vi "Text control 2 v1.3.vi"() -> ()   [LabVIEW 2016]
panel:
  in  "Serial Settings:Serial End Mode for Reads":u16(ring)=2 items=["None", "LastBit", "TermChar"]
  in  "bytes to read":u32=5
  in  "Timeout (ms)":u32=10000
  in  "Enable Termination\nChar (T)":bool=TRUE
  in  "Termination char\n(0xA = '\\n' = LF)\n(0xD = '\\r' = CR)":u8=13 format="%.0x"
  in  "flow control":u16(ring) items=["None"=0, "XON/XOFF"=1, "RTS/CTS"=2, "DTR/DSR"=4]
  in  "stop bits":u16(ring)=10 items=["1.0"=10, "1.5"=15, "2.0"=20]
  in  "parity":u16(ring) items=["None", "Odd", "Even", "Mark", "Space"]
  in  "data bits":u16=8 min=5 max=8 step=1
  in  "VISA resource name":refnum<visa-resource-name>="COM8"
  in  "baud rate":u32=9600
  out "Serial output":string
  out "error out":errorcluster
  in  "Units":bool
  out "Elapsed Time":dbl caption="Elapsed Time (s)"
  out "Ion vs time":cluster{"Y data in":dbl[], "X data in":dbl[]}[](graph)
  out "Ig":dbl format="%.2e"
  out "Id":dbl format="%.2e"
  out "Is":dbl format="%.2e"
  out "I vs Vg":cluster{"Y data in":dbl[], "X data in":dbl[]}[](graph)
  in  "Panel Controls 2":T1={"Emergency Stop"=refnum, "TransGraph Max"=1e-05, "Text/Graph (text=false)"=TRUE, "TransGraph Min"=1e-11} {"TransGraph Min" format="%.2e"; "TransGraph Max" format="%.2e"}
  out "Currently running:":string="#output s 0 0 0 -0.008 0.008 0.002"
  in  "Lines left to run:":string
  in  "Standby":T2
  in  "Full Reset":bool
  in  "SMU4":cluster{"on/off":bool, "Voltage":dbl} {"Voltage" min=-100.0 max=100.0 format="%.2f"}
  in  "Source/Drain Range":u8(slide)=6 max=11 scale=0.0..11.0
  in  "Source/Drain\nRange mode":u16(ring) items=["Auto", "Limited", "Fixed"]
  in  "Gate Range":u8(slide)=6 max=11 scale=0.0..11.0
  in  "Gate Range\nmode":u16(ring) items=["Auto", "Limited", "Fixed"]
  in  "Gate":T3={"Gate Start"=0.0, "Gate Stop"=2.0, "Gate Step (linear only)"=1.0, "Gate Compliance"=0.0001, "Gate PComp"=0.0, "Range mode"=0, "Range"=6} {"Range" max=11 scale=0.0..11.0; "Range mode" items=["Auto", "Limited", "Fixed"]; "Gate PComp" format="%^.2e"; "Gate Compliance" format="%^.2e"; "Gate Step (linear only)" format="%^.4e"; "Gate Stop" format="%^.4e"; "Gate Start" format="%^.4e"}
  in  "Drain 2":T4={"Drain Start"=0.0, "Drain Stop"=2.0, "Drain Compliance"=0.0001, "Drain Step"=1.0, "Drain PComp"=0.0, "Range mode"=0, "Range"=6} {"Range" max=11 scale=0.0..11.0; "Range mode" items=["Auto", "Limited", "Fixed"]; "Drain PComp" format="%^.2e"; "Drain Step" format="%^.4e"; "Drain Compliance" format="%^.2e"; "Drain Stop" format="%^.4e"; "Drain Start" format="%^.4e"}
  in  "Timings 2":T5={"integration time"=0, "Short/Long integration time"=0.00064, "hold time (sec)"=0.0, "delay time (sec)"=0.0, "Step Time (0 disables)"=0.0, "sweep method"=0, "Pulse period"=0.005, "Base voltage"=0.0, "Pulse width"=0.0005} {"Pulse width" min=0.0005 max=0.1 step=0.0001 format="%.4f"; "Base voltage" format="%^.4e"; "Pulse period" min=0.005 max=1.0 step=0.0001 format="%.4f"; "sweep method" items=["Continuous", "Pulsed"]; "Step Time (0 disables)" format="%.2f"; "delay time (sec)" format="%.4f"; "hold time (sec)" format="%.4f"; "Short/Long integration time" format="%^.0e"; "integration time" scale=0.0..2.0}
  in  "Panel Controls":T6={"Emergency Stop"=refnum, "TransGraph Max"=1e-05, "Text/Graph (text=false)"=TRUE} {"TransGraph Max" format="%.2e"}
  in  "Interrupt run":bool
  in  "Drain: Compliance":dbl=0.001 format="%.8f"
  in  "Gate: Compliance":dbl=0.001 format="%.8f"
  out "Path":path=path "C:/users/rlp38/09Apr2009LTtesting/test2.txt"
  in  "hold time /s":dbl format="%.2f"
  in  "delay time /s":dbl format="%.2f"
  in  "integration time":u32(slide) max=2 step=1 scale=0.0..2.0
  in  "Integration time (short)":dbl=0.0019 min=8e-05 max=0.0019 step=8e-05 format="%^.0e"
  in  "Integration time (long)":dbl=0.32 min=0.04 max=2.0 step=0.02 format="%.2f"
  in  "Step delay /s":dbl format="%.2f"
  in  "Program":string="#pulsedstressV d 0.03 20 0 0.5 0.0827 5\n#\n#itime s\n#gaterangemode l\n#drainrangemode l\n#pulsed on 0.05 0 0.02\n#transfer d 1 -1 -0.1 -1 -1 0\n#wait-min 1\n#transfer d 1 -1 -0.1 -1 -1 0\n#output d 0 -1 -0.5 0 -1 -0.1\n#transfer d -10 40 1 5 40 35\n#transfer d -10 40 1 5 40 35\n#output d 0 40 20 0 40 1\n#\n#\n#sample 1 0.008 221 6 0.003\n#samplei 400e-6 200 6 0.002 0.1\n#vsu2pulse -10 4\n#\n#stressV 0.016 0.03 2e-4 0.1e-3 11\n#stressI 220e-7 0.08 15\n#transfer s -1 1 0.5 -0.005 0.005 0.005\n#output s 0 0 0 -0.008 0.008 0.002\n"
  # "Syntax:\nitime [s|m|l]\ngaterangemode [a|l|f]\ndrainrangemode [a|l|f]\npulsed [on|off] PulsePeriod(sec) PulseBaseVoltage PulseONWidth(sec)\nstandby [on l off]\nwait NumMilliseconds\nwait-min NumMinutes\n# texthere = comment\ntransfer [s|d] VgStart VgStop VgStep VdStart VdStop VdStep\noutput [s|d] VgStart VgStop VgStep VdStart VdStop VdStep\nsample Vg Vd NumSamples Time(s) SampleInterval(s)\nsamplei Idg NumSamples Time(s) SampleInterval(s) VDGcompliance\n# if in doubt use SampleInterval(s) = 0.004\nstressV VG VD IGcompliance IDcompliance Duration(sec)\nstressI IDG VDGcompliance Duration(sec)\nvsu2pulse Bias Duration(s)\npulsedstressV [s|d] VEstop VgON VgOFF Period(s) PulseONwidth(s) Vd\nsample-fpp Vg Vd NumSamples Time\nresample-fpp Vg Vd\ntransfer-fpp [s|d] VgStart VgStop VgStep VdStart VdStop VdStep\noutput-fpp [s|d] VgStart VgStop VgStep VdStart VdStop VdStep\nserial SerialPortCommand"
  # "Time"
  # "Sec"
  # "Min"
  # "100 samples is approx 13s with medium integration"
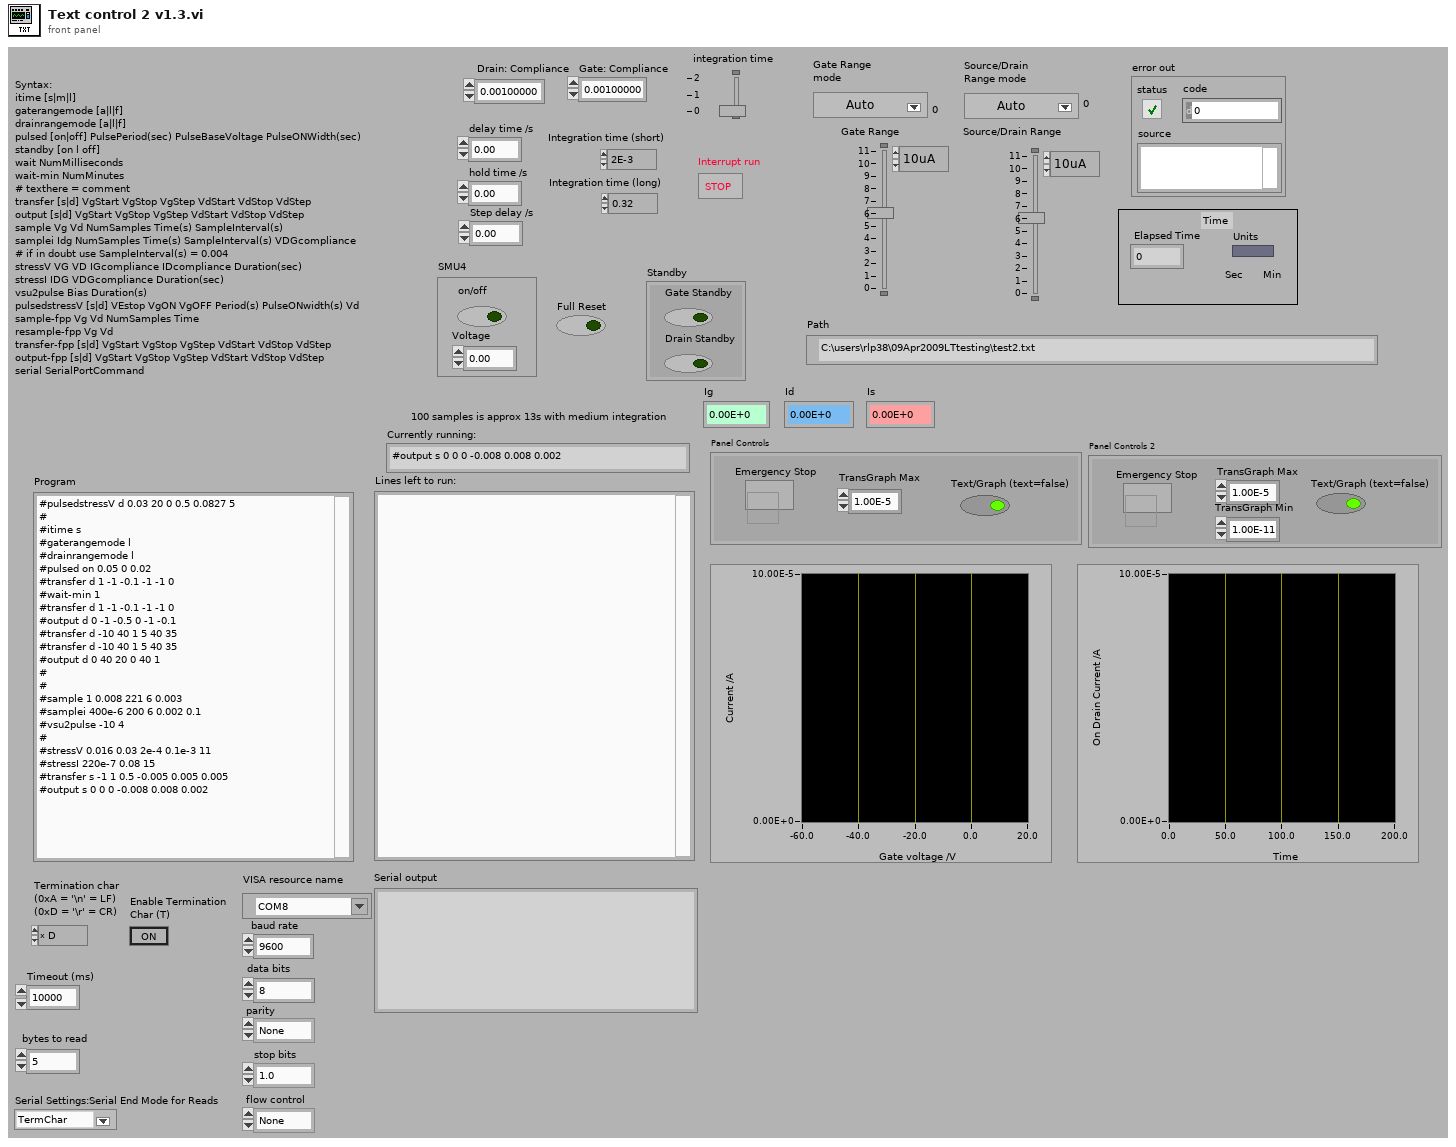
[diagram p1: front panel]
types:
  T1 = cluster{"Emergency Stop":refnum<vi>, "TransGraph Max":dbl, "Text/Graph (text=false)":bool, "TransGraph Min":dbl}
  T2 = cluster{"Gate Standby":bool, "Drain Standby":bool}
  T3 = cluster{"Gate Start":dbl, "Gate Stop":dbl, "Gate Step (linear only)":dbl, "Gate Compliance":dbl, "Gate PComp":dbl, "Range mode":u16, "Range":u8}
  T4 = cluster{"Drain Start":dbl, "Drain Stop":dbl, "Drain Compliance":dbl, "Drain Step":dbl, "Drain PComp":dbl, "Range mode":u16, "Range":u8}
  T5 = cluster{"integration time":u32, "Short/Long integration time":dbl, "hold time (sec)":dbl, "delay time (sec)":dbl, "Step Time (0 disables)":dbl, "sweep method":u16, "Pulse period":dbl, "Base voltage":dbl, "Pulse width":dbl}
  T6 = cluster{"Emergency Stop":refnum<vi>, "TransGraph Max":dbl, "Text/Graph (text=false)":bool}
  T7 = enum16{"open", "replace", "create", "open or create", "replace or create", "replace or create with confirmation"}
  T8 = cluster{"V2 Start":dbl, "V2 Step":dbl, "Number of points":i32}
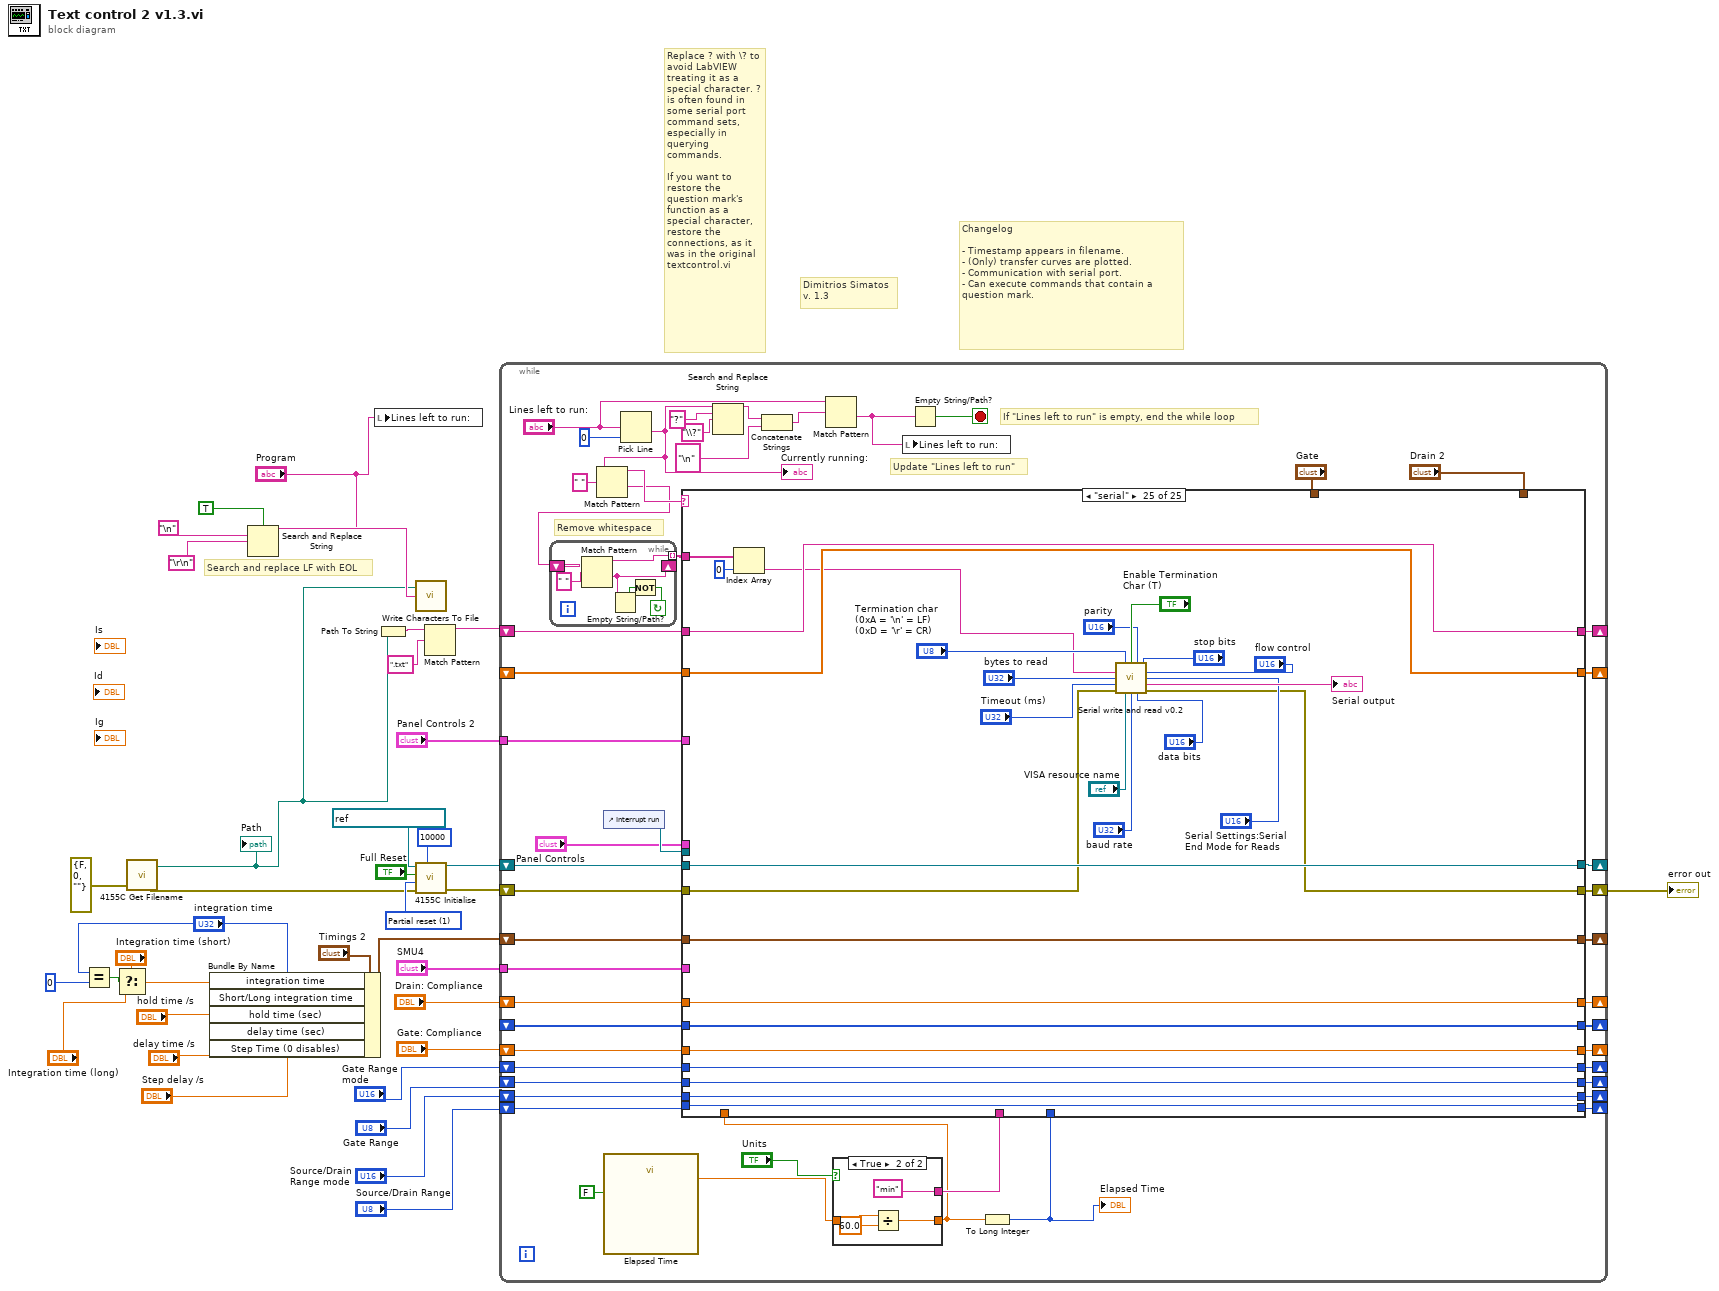
[diagram p0: block diagram]
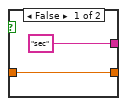
[diagram p2: hidden frame]
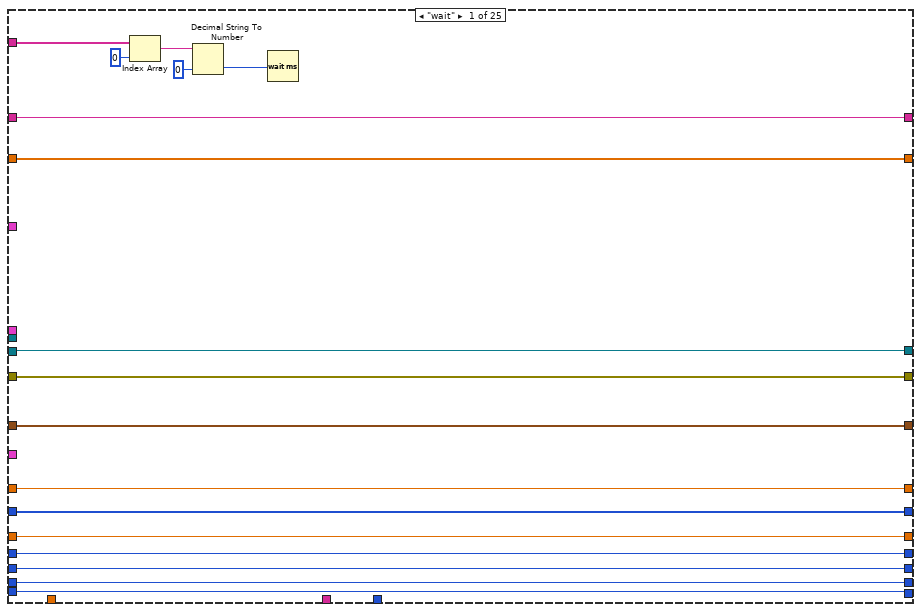
[diagram p3: hidden frame]
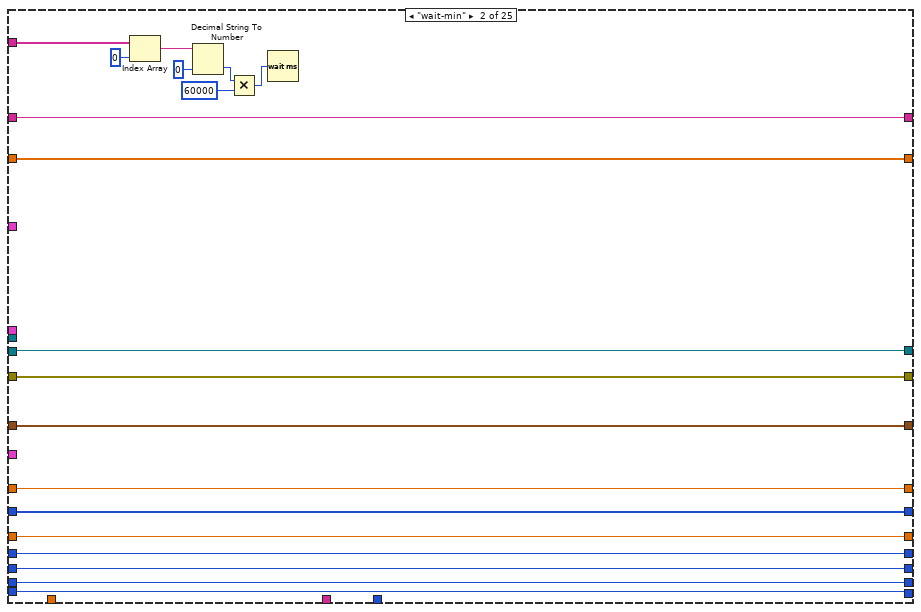
[diagram p4: hidden frame]
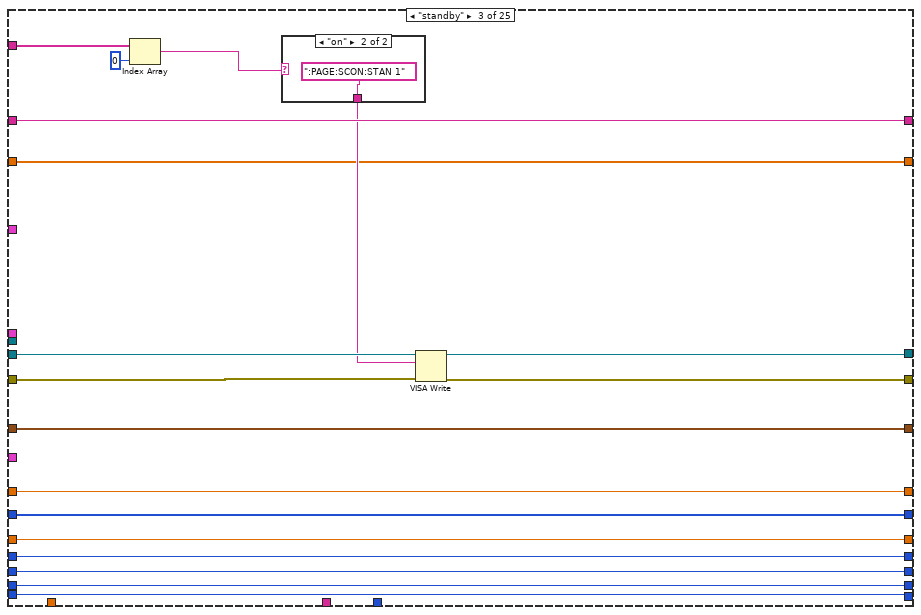
[diagram p5: hidden frame]
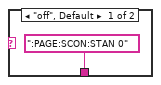
[diagram p6: hidden frame]
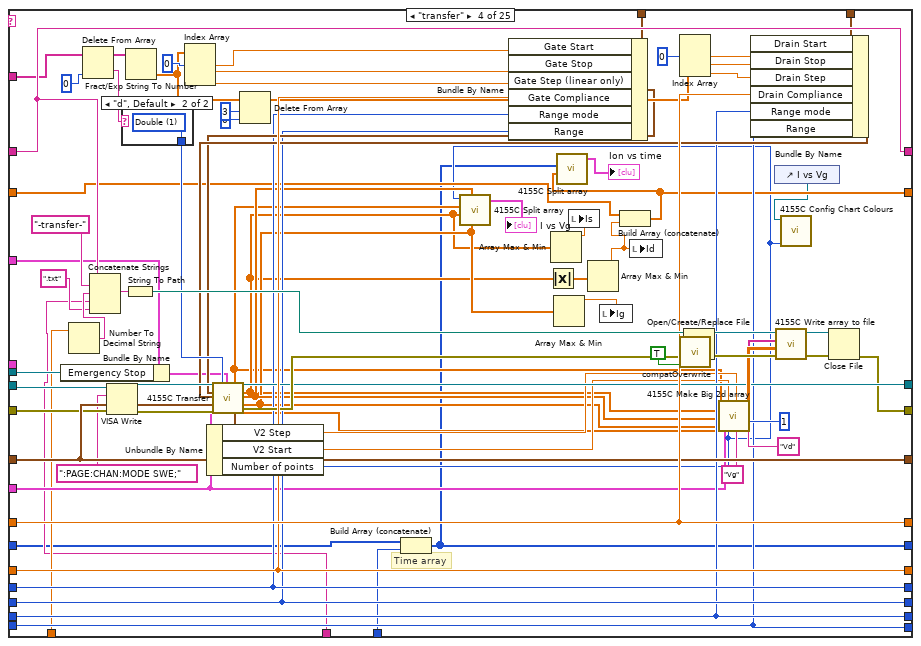
[diagram p7: hidden frame]
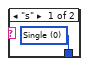
[diagram p8: hidden frame]
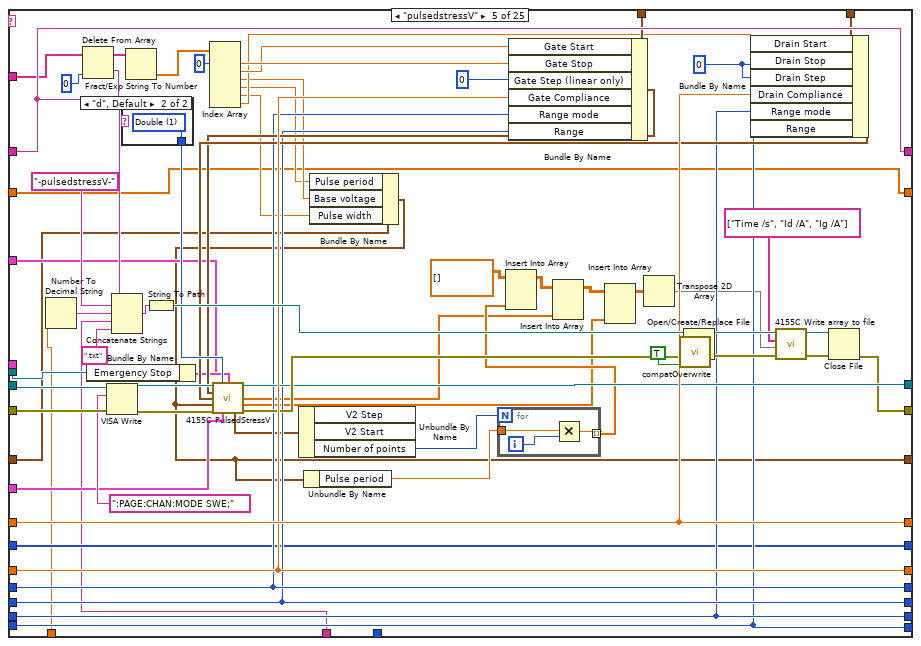
[diagram p9: hidden frame]
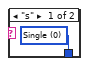
[diagram p10: hidden frame]
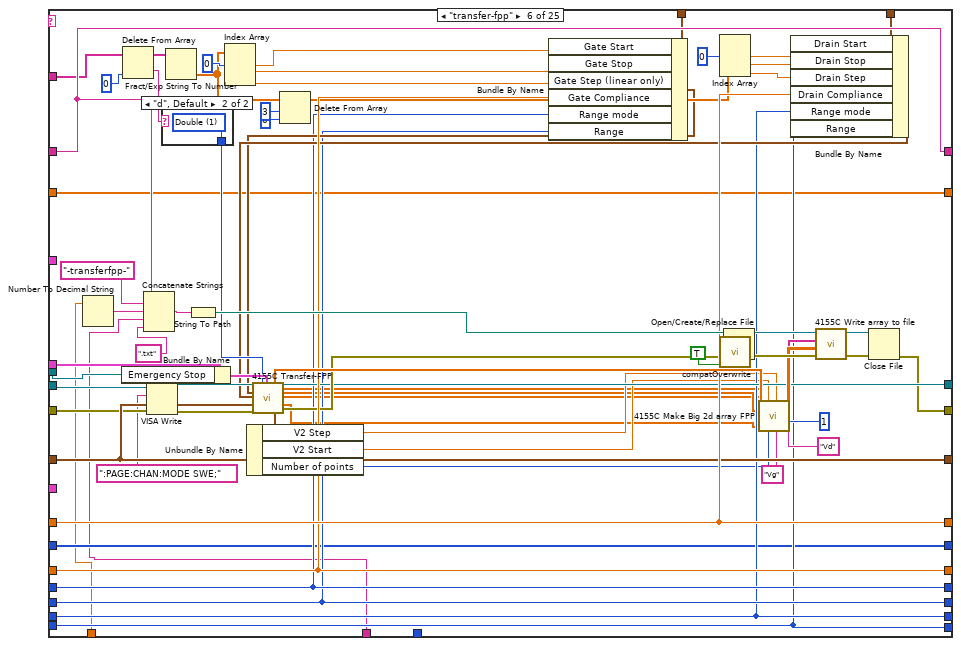
[diagram p11: hidden frame]
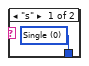
[diagram p12: hidden frame]
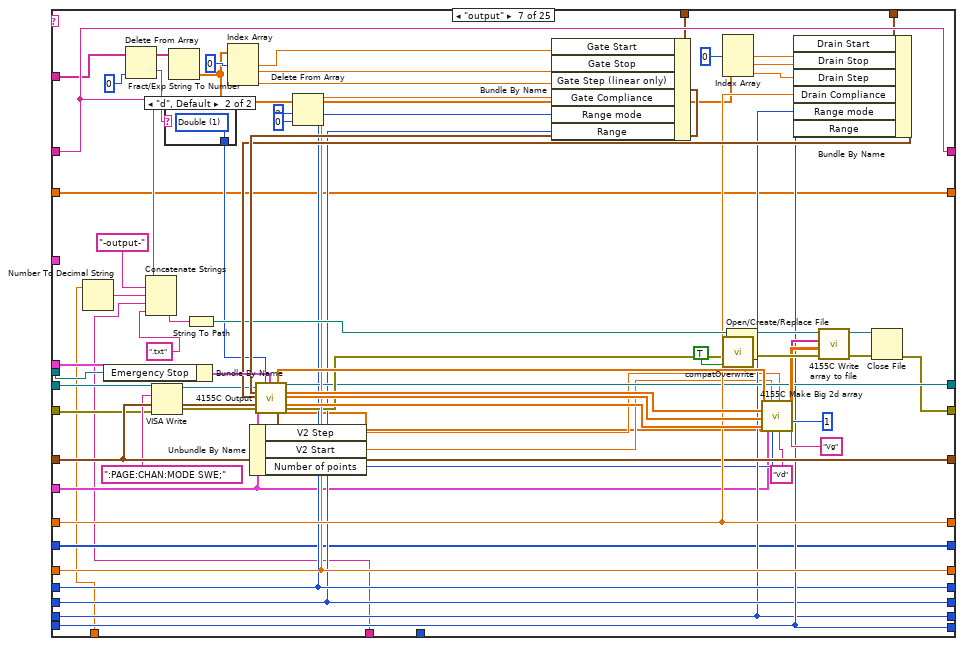
[diagram p13: hidden frame]
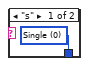
[diagram p14: hidden frame]
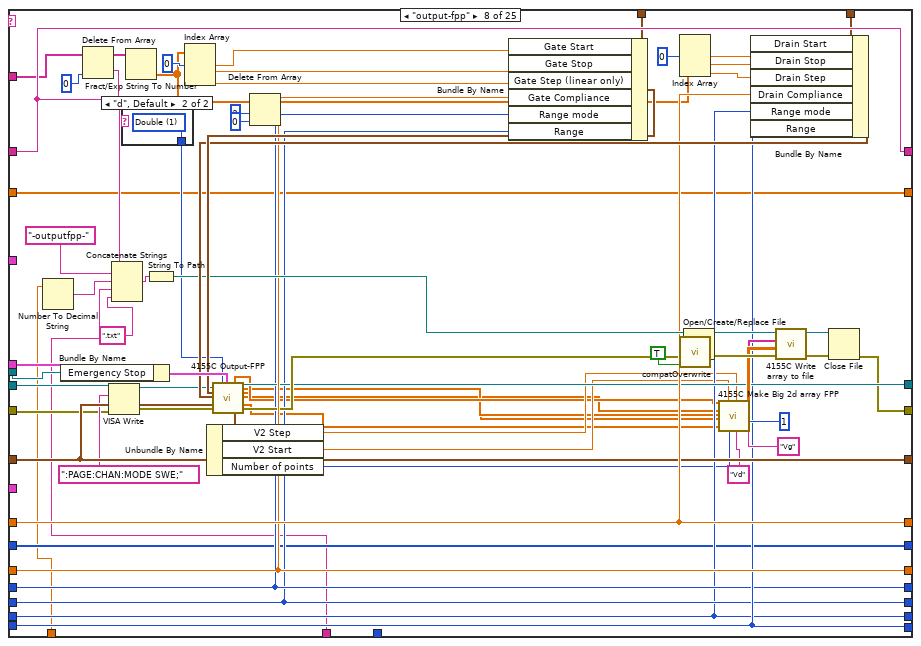
[diagram p15: hidden frame]
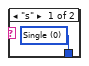
[diagram p16: hidden frame]
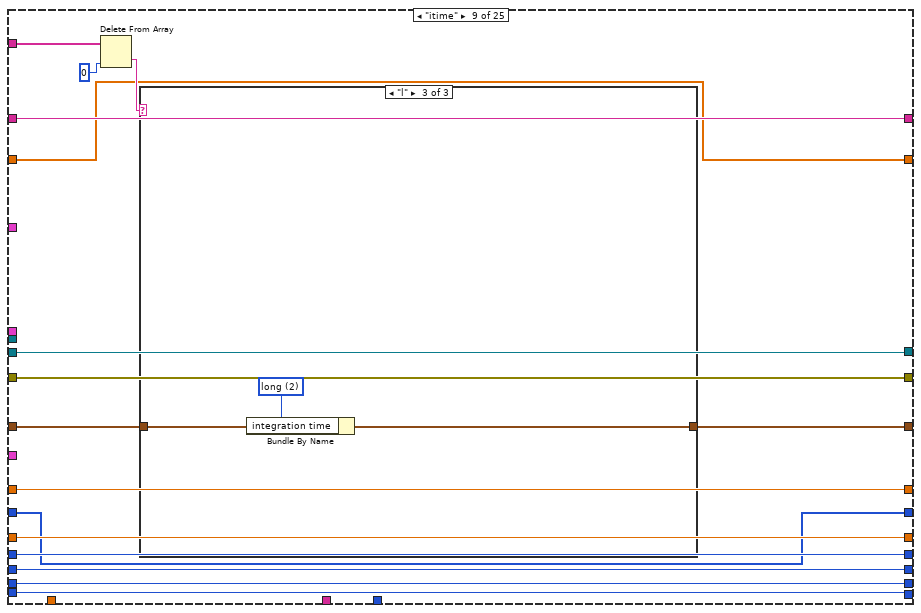
[diagram p17: hidden frame]
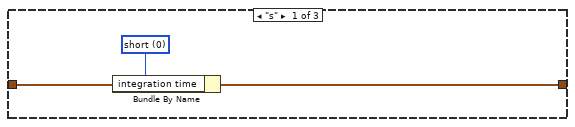
[diagram p18: hidden frame]
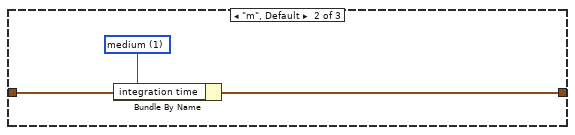
[diagram p19: hidden frame]
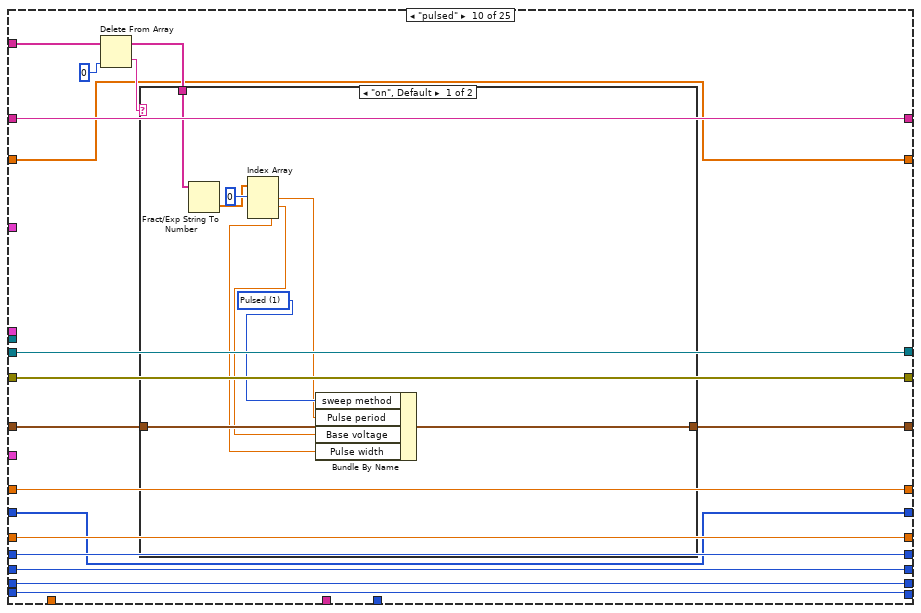
[diagram p20: hidden frame]
diagram:
  w28 = u16 1 items=["Reset All", "Partial reset"] ("Type of reset")
  # "Replace ? with \\? to avoid LabVIEW treating it as a special character. ? is often found in some serial port command sets, especially in querying commands.\n\nIf you want to restore the question mark's function as a special character, restore the connections, as it was in the original textcontrol.vi"
  # "Dimitrios Simatos\nv. 1.3"
  # "Changelog\n\n- Timestamp appears in filename.\n- (Only) transfer curves are plotted.\n- Communication with serial port.\n- Can execute commands that contain a question mark."
  # "Search and replace LF with EOL"
  n1 = Equal?(x="integration time", y=u32 0) -> (x = y?=w32:bool)
  n2 = Select(t="Integration time (short)", s=w32, f="Integration time (long)") -> (s? t:f=w36:dbl)
  n3 = call "4155C Get Filename.vi"("error in (no error)"=errorcluster {"status"=FALSE, "code"=0, "source"=""}) -> ("error out"=w23:errorcluster, "path"=w7:path)  [unwired: 2 in, 1 out]
  "Path" <- w7
  n4 = Bundle By Name(cluster="Timings 2", "integration time"="integration time", "Short/Long integration time"=w36, "hold time (sec)"="hold time /s", "delay time (sec)"="delay time /s", "Step Time (0 disables)"="Step delay /s") -> (w20:T5)
  n5 = Search and Replace String(replace all?=TRUE ("replace all? (F)"), input string="Program", search string="\n", replace string="\r\n") -> (result string=w10:string)  [unwired: 4 in, 3 out]
  n6 = local write "Lines left to run:"("Program") -> ()
  n7 = Path To String(path=w7) -> (string=w6:string)
  n8 = call <vilib>:"Write Characters To File.vi"("character string"=w10, "file path (dialog if empty)"=w7) -> ()  [unwired: 3 in, 1 out]
  n9 = call "4155C Initialise.vi"("VISA resource name in"=refnum<visa-resource-name> "GPIB0::14::INSTR", "Reset"="Full Reset", "Type of reset"=w28, "error in (no error)"=w23, "VISA Timeout Value"=u32 10000) -> ("VISA Resource Name out"=w22:refnum<visa-resource-name>, "error out"=w21:errorcluster)
  n10 = Match Pattern(string=w6, regular expression=".txt") -> (before substring=w5:string)  [unwired: 1 in, 3 out]
  n11 = while {
    tunnel: "SMU4" -> [w56]
    shift-left: "Source/Drain Range" -> [w61]
    shift-right: [w57] -> _
    shift-left: "Source/Drain\nRange mode" -> [w62]
    shift-right: [w58] -> _
    shift-left: "Gate Range" -> [w63]
    shift-right: [w59] -> _
    shift-left: "Gate Range\nmode" -> [w64]
    shift-right: [w60] -> _
    shift-left: "Gate: Compliance" -> [w75]
    shift-right: [w70] -> _
    shift-left: "Drain: Compliance" -> [w76]
    shift-right: [w71] -> _
    shift-left: w20 -> [w77]
    shift-right: [w72] -> _
    shift-left: w21 -> [w78]
    shift-right: [w73] -> w2
    shift-left: w22 -> [w79]
    shift-right: [w74] -> _
    shift-left: w5 -> [w80]
    shift-right: [w69] -> _
    tunnel: "Panel Controls 2" -> [w53]
    shift-right: [w52] -> _
    shift-left: _ -> [w51]
    shift-right: [w46] -> _
    shift-left: _ -> [w45]
    stop <- w42 stop-if-true
    # "Remove whitespace"
    # "If \"Lines left to run\" is empty, end the while loop"
    # "Update \"Lines left to run\""
    n12 = control-ref of="Interrupt run"() -> (w68:refnum<vi>)
    n13 = call "Elapsed Time"("Auto Reset"=FALSE) -> ("Elapsed Time (s)"=w47:dbl)  [unwired: 11 in, 7 out]
    n14 = Pick Line(multi-line string="Lines left to run:", line index=0) -> (output string=w41:string)  [unwired: 1 in]
    "Currently running:" <- w41
    n15 = Match Pattern(string=w41, regular expression=" ") -> (before substring=w83:string, after substring=w82:string)  [unwired: 1 in, 2 out]
    n16 = while {
      tunnel: [w94] -> w81 mode=indexing
      shift-left: w82 -> [w96]
      shift-right: [w95] -> _
      stop <- w98 continue-if-true
      n17 = Match Pattern(string=w96, regular expression=" ") -> (before substring=w94:string, after substring=w95:string)  [unwired: 1 in, 2 out]
      n18 = Empty String/Path?(string/path=w95) -> (empty?=w99:bool)
      n19 = Not(x=w99) -> (.not. x?=w98:bool)
    }
    n20 = Search and Replace String(input string=w41, search string="?", replace string="\\?") -> (result string=w39:string)  [unwired: 5 in, 3 out]
    n21 = Concatenate Strings(w39, "\n" ("Substring")) -> (w86:string)
    n22 = Match Pattern(string="Lines left to run:", regular expression=w86) -> (after substring=w54:string)  [unwired: 1 in, 3 out]
    n23 = case shown="True" "Units" {
      tunnel: ["sec" "min"] -> w48
      tunnel: [w88 w92] -> w44
      tunnel: w47 -> [w88 w91]
      frame False {
      }
      frame True {
        n24 = Divide(x=w91, y=60.0) -> (x/y=w92:dbl)
      }
    }
    n25 = local write "Lines left to run:"(w54) -> ()
    n26 = Empty String/Path?(string/path=w54) -> (empty?=w42:bool)
    n27 = To Long Integer(number=w44) -> (32bit integer=w43:i32)
    "Elapsed Time" <- w43
    n28 = case shown="\"serial\"" w83 {
      tunnel: w81 -> [w116 w135 w153 w217 w288 w357 w424 w499 w537 w563 w590 w615 w636 w650 _ _ w754 w815 _ w880 w924 w966 w1036 w1098 w1104]
      tunnel: w80 -> [w111 w131 w151 w225 w295 w365 w432 w507 w526 w552 w582 w608 w630 w643 w662 w704 w732 w797 w828 w867 w911 w954 w1030 w1094 w1106]
      tunnel: w79 -> [w110 w130 w142 w195 w279 w334 w400 w475 w527 w553 w583 w609 w631 w644 w667 w706 w760 w821 w832 w886 w930 w972 w1042 w1052 w1110]
      tunnel: w78 -> [w109 w129 w141 w194 w278 w333 w397 w472 w528 w554 w584 w610 w632 w645 w666 w677 w759 w820 w831 w885 w929 w971 w1041 w1051 w1109]
      tunnel: w77 -> [w108 w128 w150 w221 w254 w361 w428 w503 w536 w562 w581 w607 w629 w642 w665 w701 w723 w789 w837 w860 w904 w947 w1029 w1093 w1111]
      tunnel: w76 -> [w107 w127 w149 w223 w293 w363 w430 w505 w535 w561 w589 w614 w635 w649 w664 w686 w758 w819 w840 w884 w928 w970 w1040 w1102 w1112]
      tunnel: w75 -> [w106 w126 w148 w222 w292 w362 w429 w504 w534 w560 w588 w613 w634 w648 w663 w687 w733 w798 w839 w868 w912 w955 w1031 w1095 w1114]
      tunnel: [w110 w130 w140 w219 w290 w359 w426 w501 w527 w553 w583 w609 w631 w644 w667 w706 w724 w771 w830 w861 w905 w948 w982 w1054 w1110] -> w74
      tunnel: [w109 w129 w139 w218 w289 w358 w425 w500 w528 w554 w584 w610 w632 w645 w666 w676 w734 w772 w829 w869 w913 w956 w981 w1053 w1108] -> w73
      tunnel: [w108 w128 w150 w221 w250 w361 w428 w503 w529 w555 w581 w607 w629 w642 w665 w701 w723 w789 w837 w860 w904 w947 w1029 w1093 w1111] -> w72
      tunnel: [w107 w127 w149 w223 w293 w363 w430 w505 w535 w561 w589 w614 w635 w649 w664 w686 w758 w819 w840 w884 w928 w970 w1040 w1102 w1112] -> w71
      tunnel: [w106 w126 w148 w222 w292 w362 w429 w504 w534 w560 w588 w613 w634 w648 w663 w687 w733 w798 w839 w868 w912 w955 w1031 w1095 w1114] -> w70
      tunnel: [w111 w131 w151 w225 w295 w365 w432 w507 w526 w552 w582 w608 w630 w643 w662 w704 w732 w797 w828 w867 w911 w954 w1030 w1094 w1106] -> w69
      tunnel: w68 -> [_ _ _ w228 w299 w370 w440 w511 _ _ _ _ _ _ _ _ w729 w794 _ w866 w910 w953 w1002 w1070 _]
      tunnel: "Gate" -> [_ _ _ w204 w282 w344 w411 w486 _ _ _ _ _ _ _ _ _ _ _ _ _ _ _ _ _]
      tunnel: "Drain 2" -> [_ _ _ w203 w281 w343 w410 w485 _ _ _ _ _ _ _ _ _ _ _ _ _ _ _ _ _]
      tunnel: "Panel Controls" -> [_ _ _ _ _ w342 w409 w484 _ _ _ _ _ _ _ _ _ _ _ _ _ _ _ _ _]
      tunnel: w64 -> [w105 w125 w147 w188 w272 w327 w395 w470 w533 w559 _ w606 w628 w641 w661 w688 w719 w785 w833 w856 w900 w943 w1025 w1089 w1115]
      tunnel: w63 -> [w104 w124 w146 w187 w271 w326 w394 w469 w532 w558 w587 _ w619 w647 w660 w689 w720 w786 w834 w857 w901 w944 w1026 w1090 w1116]
      tunnel: w62 -> [w103 w123 w145 w186 w270 w325 w393 w468 w531 w557 w586 w612 w633 _ w659 w690 w721 w787 w835 w858 w902 w945 w1027 w1091 w1117]
      tunnel: w61 -> [w102 w122 w144 w185 w269 w324 w396 w471 w530 w556 w585 w611 _ w646 w658 w691 w722 w788 w836 w859 w903 w946 w1028 w1092 w1118]
      tunnel: [w105 w125 w147 w188 w272 w327 w395 w470 w533 w559 w580 w606 w628 w641 w661 w688 w719 w785 w833 w856 w900 w943 w1025 w1089 w1115] -> w60
      tunnel: [w104 w124 w146 w187 w271 w326 w394 w469 w532 w558 w587 w598 w619 w647 w660 w689 w720 w786 w834 w857 w901 w944 w1026 w1090 w1116] -> w59
      tunnel: [w103 w123 w145 w186 w270 w325 w393 w468 w531 w557 w586 w612 w633 w640 w659 w690 w721 w787 w835 w858 w902 w945 w1027 w1091 w1117] -> w58
      tunnel: [w102 w122 w144 w185 w269 w324 w396 w471 w530 w556 w585 w611 w620 w646 w658 w691 w722 w788 w836 w859 w903 w946 w1028 w1092 w1118] -> w57
      tunnel: w56 -> [_ _ _ w180 w266 _ w388 _ _ _ _ _ _ _ _ _ _ _ _ _ _ _ _ _ _]
      tunnel: w53 -> [_ _ _ w178 w265 _ _ _ _ _ _ _ _ _ _ _ _ _ _ _ _ _ _ _ _]
      tunnel: [w101 w118 w137 w167 w242 w314 w385 w457 w525 w550 w579 w597 w618 w639 w657 w672 w711 w769 w827 w845 w893 w937 w979 w1047 w1107] -> w52
      tunnel: w51 -> [w101 w118 w137 w166 w242 w314 w385 w457 w525 w550 w579 w597 w618 w639 w657 w672 w711 w769 w827 w845 w893 w937 w979 w1047 w1107]
      tunnel: w44 -> [_ _ _ w162 w239 w312 w382 w454 _ _ _ _ _ _ _ w670 w709 w766 _ w842 w890 w934 w976 w1043 _]
      tunnel: w48 -> [_ _ _ w159 w238 w310 w381 w453 _ _ _ _ _ _ _ w668 w707 w765 _ w841 w889 w933 w975 w1044 _]
      tunnel: w43 -> [_ _ _ w156 _ _ _ _ _ _ _ _ _ _ _ _ _ _ _ _ _ _ _ _ _]
      tunnel: [w100 w117 w136 w158 w241 w313 w384 w456 w524 w549 w578 w596 w617 w638 w656 w671 w710 w768 w826 w844 w892 w936 w978 w1046 w1113] -> w46
      tunnel: w45 -> [w100 w117 w136 w157 w241 w313 w384 w456 w524 w549 w578 w596 w617 w638 w656 w671 w710 w768 w826 w844 w892 w936 w978 w1046 w1113]
      frame "wait" {
        n29 = Index Array(array=w116, index=0 ("Index")) -> (element=w114:string)
        n30 = Decimal String To Number(string=w114, default (0L)=u32 0) -> (number=w113:u32)  [unwired: 1 in, 1 out]
        n31 = Wait (ms)(milliseconds to wait=w113) -> ()  [unwired: 1 out]
      }
      frame "wait-min" {
        n32 = Index Array(array=w135, index=0 ("Index")) -> (element=w133:string)
        n33 = Decimal String To Number(string=w133, default (0L)=u32 0) -> (number=w121:u32)  [unwired: 1 in, 1 out]
        n34 = Multiply(x=w121, y=u32 60000) -> (x*y=w120:u32)
        n35 = Wait (ms)(milliseconds to wait=w120) -> ()  [unwired: 1 out]
      }
      frame "standby" {
        n36 = Index Array(array=w153, index=0 ("Index")) -> (element=w143:string)
        n37 = case shown="\"on\"" w143 {
          tunnel: [":PAGE:SCON:STAN 0" ":PAGE:SCON:STAN 1"] -> w138
          frame "off", Default {
          }
          frame "on" {
          }
        }
        n38 = VISA Write(VISA resource name=w142, write buffer=w138, error in (no error)=w141) -> (VISA resource name out=w140:refnum<visa-resource-name>, error out=w139:errorcluster)  [unwired: 1 out]
      }
      frame "transfer" {
        # "Time array"
        n39 = Bundle By Name(cluster=w178, "Emergency Stop"=w228) -> (w179:T1)
        n40 = Number To Decimal String(number=w162) -> (decimal integer string=w161:string)  [unwired: 1 in]
        n41 = Delete From Array(array=w217, index=0 ("Index")) -> (deleted portion=w215:string, array with subset deleted=w214:string[])  [unwired: 1 in]
        n42 = Concatenate Strings(w225, "-transfer-" ("Prefix"), w161, w159, ".txt" ("Suffix")) -> (w227:string)
        n43 = VISA Write(VISA resource name=w195, write buffer=":PAGE:CHAN:MODE SWE;" ("write buffer (\"\")"), error in (no error)=w194) -> (VISA resource name out=w192:refnum<visa-resource-name>, error out=w193:errorcluster)  [unwired: 1 out]
        n44 = case shown="\"d\", Default" w215 {
          tunnel: [w236 w237] -> w213
          frame "s" {
            w236 = u16 0 items=["Single", "Double"] ("sweep mode")
          }
          frame "d", Default {
            w237 = u16 1 items=["Single", "Double"] ("sweep mode")
          }
        }
        n45 = String To Path(string=w227) -> (path=w224:path)
        n46 = Fract/Exp String To Number(string=w214) -> (number=w199:dbl[])  [unwired: 3 in, 1 out]
        n47 = Index Array(array=w199, index #1=0 ("Index")) -> (element #1=w212:dbl, element #2=w211:dbl, element #3=w210:dbl)  [unwired: 2 in]
        n48 = Delete From Array(array=w199, length=3 ("Length"), index=0 ("Index")) -> (array with subset deleted=w197:dbl[])  [unwired: 1 out]
        n49 = Build Array (concatenate)(w157, w156) -> (w158:i32[])
        n50 = Bundle By Name(cluster=w204, "Gate Start"=w212, "Gate Stop"=w211, "Gate Step (linear only)"=w210, "Gate Compliance"=w222, "Range mode"=w188, "Range"=w187) -> (w189:T3)
        n51 = Index Array(array=w197, index #1=0 ("Index")) -> (element #1=w207:dbl, element #2=w206:dbl, element #3=w205:dbl)  [unwired: 2 in]
        n52 = call <vilib>:"compatOverwrite.vi"("overwrite (F)"=TRUE) -> ("overwrite?"=w177:T7)
        n53 = Bundle By Name(cluster=w203, "Drain Start"=w207, "Drain Stop"=w206, "Drain Step"=w205, "Drain Compliance"=w223, "Range mode"=w186, "Range"=w185) -> (w190:T4)
        n54 = call "4155C Transfer.vi"("VISA resource name in"=w192, "Gate"=w189, "Drain"=w190, "Timings"=w221, "error in (no error)"=w193, "SMU4"=w180, "sweep mode"=w213, "Panel Controls"=w179) -> ("VG"=w168:dbl[], "Outparams"=w184:T8, "VISA Resource Name out"=w219:refnum<visa-resource-name>, "IS"=w170:dbl[], "ID"=w175:dbl[], "IG"=w171:dbl[], "error out"=w220:errorcluster, "SMU4"=w181:dbl[])  [unwired: 12 in]
        n55 = Unbundle By Name(w184) -> ("V2 Step"=w183:dbl, "V2 Start"=w182:dbl, "Number of points"=w164:i32)
        n56 = call "4155C Split array.vi"("Number of VAR2 steps"=w164, "Y2 data in"=w175, "X data in"=w168, "Y1 data in"=w170, "Y3 data in"=w171) -> ("Array of clusters"=→"I vs Vg":cluster{"Y data in":dbl[], "X data in":dbl[]}[])  [unwired: 2 in, 1 out]
        n57 = Absolute Value(x=w170) -> (abs(x)=w174:dbl[])
        n58 = Array Max & Min(array=w170) -> (max value=w172:dbl)  [unwired: 3 out]
        n59 = Array Max & Min(array=w171) -> (max value=w173:dbl)  [unwired: 3 out]
        n60 = local write "Is"(w172) -> ()
        n61 = Array Max & Min(array=w174) -> (max value=w165:dbl)  [unwired: 3 out]
        n62 = local write "Ig"(w173) -> ()
        n63 = Build Array (concatenate)(w166, w165) -> (w167:dbl[])
        n64 = call "4155C Split array.vi"("X data in"=w158, "Y1 data in"=w167) -> ("Array of clusters"=→"Ion vs time":cluster{"Y data in":dbl[], "X data in":dbl[]}[])  [unwired: 5 in, 1 out]
        n65 = local write "Id"(w165) -> ()
        n66 = Open/Create/Replace File(file path (use dialog)=w224, error in=w220, operation (0:open)=w177) -> (refnum out=w233:refnum<file>, error out=w234:errorcluster)  [unwired: 3 in, 1 out]
        n67 = call "4155C Make Big 2d array.vi"("1D Var1"=w168, "1d IS"=w170, "1d ID"=w175, "1d IG"=w171, "1d SMU4"=w181, "SMU4"=w180, "VAR2 START"=w182, "Number of VAR2 steps"=w164, "VAR2 STEP"=w183, "VAR1 Name"="Vg", "Decimal places in header"=i8 1, "VAR2 Name"="Vd") -> ("Header array"=w229:string[], "Data array"=w230:dbl[][])  [unwired: 14 in]
        n68 = control-ref of="I vs Vg"() -> (w163:refnum<vi>)
        n69 = call "4155C Write array to file.vi"("Byte Stream File Refnum"=w233, "Header"=w229, "Data Array"=w230, "error in (no error)"=w234) -> ("dup refnum"=w231:refnum<file>, "error out"=w232:errorcluster)  [unwired: 1 in]
        n70 = call "4155C Config Chart Colours.vi"("Numeric"=w164, "XY Graph 2"=w163) -> ()  [unwired: 6 in]
        n71 = Close File(refnum=w231, error in=w232) -> (error out=w218:errorcluster)  [unwired: 1 out]
      }
      frame "pulsedstressV" {
        w248 = 0
        n72 = Number To Decimal String(number=w239) -> (decimal integer string=w296:string)  [unwired: 1 in]
        n73 = Delete From Array(array=w288, index=0 ("Index")) -> (deleted portion=w286:string, array with subset deleted=w285:string[])  [unwired: 1 in]
        n74 = Bundle By Name(cluster=w265, "Emergency Stop"=w299) -> (w267:T1)
        n75 = VISA Write(VISA resource name=w279, write buffer=":PAGE:CHAN:MODE SWE;" ("write buffer (\"\")"), error in (no error)=w278) -> (VISA resource name out=w276:refnum<visa-resource-name>, error out=w277:errorcluster)  [unwired: 1 out]
        n76 = Concatenate Strings(w295, "-pulsedstressV-" ("Substring"), w296, w238, ".txt" ("Substring")) -> (w298:string)
        n77 = case shown="\"d\", Default" w286 {
          tunnel: [w308 w309] -> w284
          frame "s" {
            w308 = u16 0 items=["Single", "Double"] ("sweep mode")
          }
          frame "d", Default {
            w309 = u16 1 items=["Single", "Double"] ("sweep mode")
          }
        }
        n78 = Fract/Exp String To Number(string=w285) -> (number=w280:dbl[])  [unwired: 3 in, 1 out]
        n79 = String To Path(string=w298) -> (path=w294:path)
        n80 = Index Array(array=w280, index #1=0 ("Index")) -> (element #1=w257:dbl, element #2=w256:dbl, element #3=w253:dbl, element #4=w252:dbl, element #5=w251:dbl, element #6=w255:dbl)  [unwired: 5 in]
        n81 = Bundle By Name(cluster=w254, "Pulse period"=w252, "Base voltage"=w253, "Pulse width"=w251) -> (w250:T5)
        n82 = Unbundle By Name(w250) -> ("Pulse period"=w258:dbl)
        n83 = Bundle By Name(cluster=w282, "Gate Start"=w256, "Gate Stop"=w257, "Gate Step (linear only)"=0, "Gate Compliance"=w292, "Range mode"=w272, "Range"=w271) -> (w273:T3)
        n84 = call <vilib>:"compatOverwrite.vi"("overwrite (F)"=TRUE) -> ("overwrite?"=w243:T7)
        n85 = Bundle By Name(cluster=w281, "Drain Start"=w255, "Drain Stop"=w248, "Drain Step"=w248, "Drain Compliance"=w293, "Range mode"=w270, "Range"=w269) -> (w274:T4)
        n86 = call "4155C PulsedStressV.vi"("VISA resource name in"=w276, "sweep mode"=w284, "Panel Controls"=w267, "Gate"=w273, "Drain"=w274, "Timings"=w250, "error in (no error)"=w277, "SMU4"=w266) -> ("VISA Resource Name out"=w290:refnum<visa-resource-name>, "ID"=w246:dbl[], "IG"=w244:dbl[], "Outparams"=w268:T8, "error out"=w291:errorcluster)  [unwired: 3 in]
        n87 = Unbundle By Name(w268) -> ("Number of points"=w245:i32)  [unwired: 2 out]
        n88 = for {
          N: w245 -> [_]
          tunnel: [w305] -> w247 mode=indexing
          tunnel: w258 -> [w307]
          i -> [w306]
          n89 = Multiply(x=w307, y=w306) -> (x*y=w305:dbl)
        }
        n90 = Insert Into Array(array=dbl[][] [] ("Input Array"), new element=w247) -> (w259:dbl[][])  [unwired: 2 in]
        n91 = Insert Into Array(array=w259, new element=w246) -> (w264:dbl[][])  [unwired: 2 in]
        n92 = Insert Into Array(array=w264, new element=w244) -> (w263:dbl[][])  [unwired: 2 in]
        n93 = Transpose 2D Array(2D array=w263) -> (transposed array=w262:dbl[][])
        n94 = Open/Create/Replace File(file path (use dialog)=w294, error in=w291, operation (0:open)=w243) -> (refnum out=w302:refnum<file>, error out=w303:errorcluster)  [unwired: 3 in, 1 out]
        n95 = call "4155C Write array to file.vi"("Byte Stream File Refnum"=w302, "Header"=string[] ["Time /s", "Id /A", "Ig /A"], "Data Array"=w262, "error in (no error)"=w303) -> ("dup refnum"=w300:refnum<file>, "error out"=w301:errorcluster)  [unwired: 1 in]
        n96 = Close File(refnum=w300, error in=w301) -> (error out=w289:errorcluster)  [unwired: 1 out]
      }
      frame "transfer-fpp" {
        n97 = Number To Decimal String(number=w312) -> (decimal integer string=w366:string)  [unwired: 1 in]
        n98 = Bundle By Name(cluster=w342, "Emergency Stop"=w370) -> (w378:T6)
        n99 = Delete From Array(array=w357, index=0 ("Index")) -> (deleted portion=w355:string, array with subset deleted=w354:string[])  [unwired: 1 in]
        n100 = Concatenate Strings(w365, "-transferfpp-" ("Substring"), w366, w310, ".txt" ("Substring")) -> (w368:string)
        n101 = VISA Write(VISA resource name=w334, write buffer=":PAGE:CHAN:MODE SWE;" ("write buffer (\"\")"), error in (no error)=w333) -> (VISA resource name out=w331:refnum<visa-resource-name>, error out=w332:errorcluster)  [unwired: 1 out]
        n102 = case shown="\"d\", Default" w355 {
          tunnel: [w379 w380] -> w353
          frame "s" {
            w379 = u16 0 items=["Single", "Double"] ("sweep mode")
          }
          frame "d", Default {
            w380 = u16 1 items=["Single", "Double"] ("sweep mode")
          }
        }
        n103 = Fract/Exp String To Number(string=w354) -> (number=w338:dbl[])  [unwired: 3 in, 1 out]
        n104 = String To Path(string=w368) -> (path=w364:path)
        n105 = Index Array(array=w338, index #1=0 ("Index")) -> (element #1=w352:dbl, element #2=w351:dbl, element #3=w350:dbl)  [unwired: 2 in]
        n106 = Delete From Array(array=w338, length=3 ("Length"), index=0 ("Index")) -> (array with subset deleted=w336:dbl[])  [unwired: 1 out]
        n107 = Bundle By Name(cluster=w344, "Gate Start"=w352, "Gate Stop"=w351, "Gate Step (linear only)"=w350, "Gate Compliance"=w362, "Range mode"=w327, "Range"=w326) -> (w328:T3)
        n108 = Index Array(array=w336, index #1=0 ("Index")) -> (element #1=w347:dbl, element #2=w346:dbl, element #3=w345:dbl)  [unwired: 2 in]
        n109 = call <vilib>:"compatOverwrite.vi"("overwrite (F)"=TRUE) -> ("overwrite?"=w315:T7)
        n110 = Bundle By Name(cluster=w343, "Drain Start"=w347, "Drain Stop"=w346, "Drain Step"=w345, "Drain Compliance"=w363, "Range mode"=w325, "Range"=w324) -> (w329:T4)
        n111 = call "4155C Transfer-FPP.vi"("VISA resource name in"=w331, "Gate"=w328, "Drain"=w329, "Timings"=w361, "error in (no error)"=w332, "sweep mode"=w353, "Panel Controls"=w378) -> ("VG"=w369:dbl[], "Outparams"=w323:T8, "VISA Resource Name out"=w359:refnum<visa-resource-name>, "Vprobe2"=w319:dbl[], "ID"=w318:dbl[], "IG"=w317:dbl[], "Vprobe1"=w316:dbl[], "error out"=w360:errorcluster)  [unwired: 13 in]
        n112 = Unbundle By Name(w323) -> ("V2 Step"=w322:dbl, "V2 Start"=w321:dbl, "Number of points"=w320:i32)
        n113 = Open/Create/Replace File(file path (use dialog)=w364, error in=w360, operation (0:open)=w315) -> (refnum out=w375:refnum<file>, error out=w376:errorcluster)  [unwired: 3 in, 1 out]
        n114 = call "4155C Make Big 2d array FPP.vi"("1D Var1"=w369, "1d ID"=w318, "1d Vp2"=w319, "1d IG"=w317, "1d Vp1"=w316, "VAR2 START"=w321, "Number of VAR2 steps"=w320, "VAR2 STEP"=w322, "VAR1 Name"="Vg", "Decimal places in header"=i8 1, "VAR2 Name"="Vd") -> ("Header array"=w371:string[], "Data array"=w372:dbl[][])  [unwired: 15 in]
        n115 = call "4155C Write array to file.vi"("Byte Stream File Refnum"=w375, "Header"=w371, "Data Array"=w372, "error in (no error)"=w376) -> ("dup refnum"=w373:refnum<file>, "error out"=w374:errorcluster)  [unwired: 1 in]
        n116 = Close File(refnum=w373, error in=w374) -> (error out=w358:errorcluster)  [unwired: 1 out]
      }
      frame "output" {
        n117 = Number To Decimal String(number=w382) -> (decimal integer string=w433:string)  [unwired: 1 in]
        n118 = Bundle By Name(cluster=w409, "Emergency Stop"=w440) -> (w450:T6)
        n119 = Delete From Array(array=w424, index=0 ("Index")) -> (deleted portion=w422:string, array with subset deleted=w421:string[])  [unwired: 1 in]
        n120 = Concatenate Strings(w432, "-output-" ("Substring"), w433, w381, ".txt" ("Substring")) -> (w435:string)
        n121 = VISA Write(VISA resource name=w400, write buffer=":PAGE:CHAN:MODE SWE;" ("write buffer (\"\")"), error in (no error)=w397) -> (VISA resource name out=w399:refnum<visa-resource-name>, error out=w398:errorcluster)  [unwired: 1 out]
        n122 = case shown="\"d\", Default" w422 {
          tunnel: [w451 w452] -> w420
          frame "s" {
            w451 = u16 0 items=["Single", "Double"] ("sweep mode")
          }
          frame "d", Default {
            w452 = u16 1 items=["Single", "Double"] ("sweep mode")
          }
        }
        n123 = Fract/Exp String To Number(string=w421) -> (number=w403:dbl[])  [unwired: 3 in, 1 out]
        n124 = String To Path(string=w435) -> (path=w431:path)
        n125 = Index Array(array=w403, index #1=0 ("Index")) -> (element #1=w419:dbl, element #2=w418:dbl, element #3=w417:dbl)  [unwired: 2 in]
        n126 = Delete From Array(array=w403, length=3 ("Length"), index=0 ("Index")) -> (array with subset deleted=w402:dbl[])  [unwired: 1 out]
        n127 = Bundle By Name(cluster=w411, "Gate Start"=w419, "Gate Stop"=w418, "Gate Step (linear only)"=w417, "Gate Compliance"=w429, "Range mode"=w395, "Range"=w394) -> (w449:T3)
        n128 = Index Array(array=w402, index #1=0 ("Index")) -> (element #1=w414:dbl, element #2=w413:dbl, element #3=w412:dbl)  [unwired: 2 in]
        n129 = call <vilib>:"compatOverwrite.vi"("overwrite (F)"=TRUE) -> ("overwrite?"=w386:T7)
        n130 = Bundle By Name(cluster=w410, "Drain Start"=w414, "Drain Stop"=w413, "Drain Step"=w412, "Drain Compliance"=w430, "Range mode"=w393, "Range"=w396) -> (w448:T4)
        n131 = call "4155C Output.vi"("VISA resource name in"=w399, "Gate"=w449, "Drain"=w448, "Timings"=w428, "error in (no error)"=w398, "SMU4"=w388, "sweep mode"=w420, "Panel controls"=w450) -> ("VD"=w436:dbl[], "Outparams"=w391:T8, "VISA Resource Name out"=w426:refnum<visa-resource-name>, "IS"=w439:dbl[], "ID"=w438:dbl[], "IG"=w437:dbl[], "error out"=w427:errorcluster, "SMU4"=w387:dbl[])  [unwired: 12 in]
        n132 = Unbundle By Name(w391) -> ("V2 Step"=w392:dbl, "V2 Start"=w390:dbl, "Number of points"=w389:i32)
        n133 = Open/Create/Replace File(file path (use dialog)=w431, error in=w427, operation (0:open)=w386) -> (refnum out=w445:refnum<file>, error out=w446:errorcluster)  [unwired: 3 in, 1 out]
        n134 = call "4155C Make Big 2d array.vi"("1D Var1"=w436, "1d IS"=w439, "1d ID"=w438, "1d IG"=w437, "1d SMU4"=w387, "SMU4"=w388, "VAR2 START"=w390, "Number of VAR2 steps"=w389, "VAR2 STEP"=w392, "VAR1 Name"="Vd", "Decimal places in header"=i8 1, "VAR2 Name"="Vg") -> ("Header array"=w441:string[], "Data array"=w442:dbl[][])  [unwired: 14 in]
        n135 = call "4155C Write array to file.vi"("Byte Stream File Refnum"=w445, "Header"=w441, "Data Array"=w442, "error in (no error)"=w446) -> ("dup refnum"=w443:refnum<file>, "error out"=w444:errorcluster)  [unwired: 1 in]
        n136 = Close File(refnum=w443, error in=w444) -> (error out=w425:errorcluster)  [unwired: 1 out]
      }
      frame "output-fpp" {
        n137 = Number To Decimal String(number=w454) -> (decimal integer string=w508:string)  [unwired: 1 in]
        n138 = Bundle By Name(cluster=w484, "Emergency Stop"=w511) -> (w521:T6)
        n139 = Delete From Array(array=w499, index=0 ("Index")) -> (deleted portion=w497:string, array with subset deleted=w496:string[])  [unwired: 1 in]
        n140 = VISA Write(VISA resource name=w475, write buffer=":PAGE:CHAN:MODE SWE;" ("write buffer (\"\")"), error in (no error)=w472) -> (VISA resource name out=w474:refnum<visa-resource-name>, error out=w473:errorcluster)  [unwired: 1 out]
        n141 = Concatenate Strings(w507, "-outputfpp-" ("Substring"), w508, w453, ".txt" ("Substring")) -> (w510:string)
        n142 = case shown="\"d\", Default" w497 {
          tunnel: [w522 w523] -> w495
          frame "s" {
            w522 = u16 0 items=["Single", "Double"] ("sweep mode")
          }
          frame "d", Default {
            w523 = u16 1 items=["Single", "Double"] ("sweep mode")
          }
        }
        n143 = Fract/Exp String To Number(string=w496) -> (number=w478:dbl[])  [unwired: 3 in, 1 out]
        n144 = String To Path(string=w510) -> (path=w506:path)
        n145 = Index Array(array=w478, index #1=0 ("Index")) -> (element #1=w494:dbl, element #2=w493:dbl, element #3=w492:dbl)  [unwired: 2 in]
        n146 = Delete From Array(array=w478, length=3 ("Length"), index=0 ("Index")) -> (array with subset deleted=w477:dbl[])  [unwired: 1 out]
        n147 = Bundle By Name(cluster=w486, "Gate Start"=w494, "Gate Stop"=w493, "Gate Step (linear only)"=w492, "Gate Compliance"=w504, "Range mode"=w470, "Range"=w469) -> (w520:T3)
        n148 = Index Array(array=w477, index #1=0 ("Index")) -> (element #1=w489:dbl, element #2=w488:dbl, element #3=w487:dbl)  [unwired: 2 in]
        n149 = call <vilib>:"compatOverwrite.vi"("overwrite (F)"=TRUE) -> ("overwrite?"=w458:T7)
        n150 = Bundle By Name(cluster=w485, "Drain Start"=w489, "Drain Stop"=w488, "Drain Step"=w487, "Drain Compliance"=w505, "Range mode"=w468, "Range"=w471) -> (w519:T4)
        n151 = call "4155C Output-FPP.vi"("VISA resource name in"=w474, "Gate"=w520, "Drain"=w519, "Timings"=w503, "error in (no error)"=w473, "sweep mode"=w495, "Panel controls"=w521) -> ("VD"=w463:dbl[], "Outparams"=w466:T8, "VISA Resource Name out"=w501:refnum<visa-resource-name>, "Vprobe2"=w462:dbl[], "ID"=w461:dbl[], "IG"=w460:dbl[], "Vprobe1"=w459:dbl[], "error out"=w502:errorcluster)  [unwired: 13 in]
        n152 = Unbundle By Name(w466) -> ("V2 Step"=w467:dbl, "V2 Start"=w465:dbl, "Number of points"=w464:i32)
        n153 = Open/Create/Replace File(file path (use dialog)=w506, error in=w502, operation (0:open)=w458) -> (refnum out=w516:refnum<file>, error out=w517:errorcluster)  [unwired: 3 in, 1 out]
        n154 = call "4155C Make Big 2d array FPP.vi"("1D Var1"=w463, "1d ID"=w461, "1d Vp2"=w462, "1d IG"=w460, "1d Vp1"=w459, "VAR2 START"=w465, "Number of VAR2 steps"=w464, "VAR2 STEP"=w467, "VAR1 Name"="Vd", "Decimal places in header"=i8 1, "VAR2 Name"="Vg") -> ("Header array"=w512:string[], "Data array"=w513:dbl[][])  [unwired: 15 in]
        n155 = call "4155C Write array to file.vi"("Byte Stream File Refnum"=w516, "Header"=w512, "Data Array"=w513, "error in (no error)"=w517) -> ("dup refnum"=w514:refnum<file>, "error out"=w515:errorcluster)  [unwired: 1 in]
        n156 = Close File(refnum=w514, error in=w515) -> (error out=w500:errorcluster)  [unwired: 1 out]
      }
      frame "itime" {
        n157 = Delete From Array(array=w537, index=0 ("Index")) -> (deleted portion=w538:string)  [unwired: 1 in, 1 out]
        n158 = case shown="\"l\"" w538 {
          tunnel: w536 -> [w542 w544 w547]
          tunnel: [w541 w543 w546] -> w529
          frame "s" {
            w540 = u32 0 items=["short  ", "medium  ", "long  "] ("integration time 2")
            n159 = Bundle By Name(cluster=w542, "integration time"=w540) -> (w541:T5)
          }
          frame "m", Default {
            w545 = u32 1 items=["short  ", "medium  ", "long  "] ("integration time 2")
            n160 = Bundle By Name(cluster=w544, "integration time"=w545) -> (w543:T5)
          }
          frame "l" {
            w548 = u32 2 items=["short  ", "medium  ", "long  "] ("integration time 2")
            n161 = Bundle By Name(cluster=w547, "integration time"=w548) -> (w546:T5)
          }
        }
      }
      frame "pulsed" {
        n162 = Delete From Array(array=w563, index=0 ("Index")) -> (deleted portion=w564:string, array with subset deleted=w551:string[])  [unwired: 1 in]
        n163 = case shown="\"on\", Default" w564 {
          tunnel: w562 -> [w574 w577]
          tunnel: [w573 w576] -> w555
          tunnel: w551 -> [w571 _]
          frame "on", Default {
            w572 = u16 1 items=["Continuous", "Pulsed"] ("sweep method")
            n164 = Fract/Exp String To Number(string=w571) -> (number=w569:dbl[])  [unwired: 3 in, 1 out]
            n165 = Index Array(array=w569, index #1=0 ("Index")) -> (element #1=w568:dbl, element #2=w567:dbl, element #3=w566:dbl)  [unwired: 2 in]
            n166 = Bundle By Name(cluster=w574, "sweep method"=w572, "Pulse period"=w568, "Base voltage"=w567, "Pulse width"=w566) -> (w573:T5)
          }
          frame "off" {
            w575 = u16 0 items=["Continuous", "Pulsed"] ("sweep method")
            n167 = Bundle By Name(cluster=w577, "sweep method"=w575) -> (w576:T5)
          }
        }
      }
      frame "gaterangemode" {
        n168 = Delete From Array(array=w590, index=0 ("Index")) -> (deleted portion=w591:string)  [unwired: 1 in, 1 out]
        n169 = case shown="\"f\"" w591 {
          tunnel: [w593 w594 w595] -> w580
          frame "a", Default {
            w593 = u16 0 items=["Auto", "Limited", "Fixed"] ("Gate Range\nmode 2")
          }
          frame "f" {
            w594 = u16 2 items=["Auto", "Limited", "Fixed"] ("Gate Range\nmode 2")
          }
          frame "l" {
            w595 = u16 1 items=["Auto", "Limited", "Fixed"] ("Gate Range\nmode 2")
          }
        }
      }
      frame "gaterange" {
        (unwired) u8 11 items=["10fA  ", "100fA  ", "1nA  ", "10nA", "100nA", "1uA", "10uA", "100uA", "1mA", "10mA", "100mA", "1A"] ("Gate Range 2")
        n170 = Delete From Array(array=w615, index=0 ("Index")) -> (deleted portion=w605:string)  [unwired: 1 in, 1 out]
        n171 = Scan Value(string=w605, format string="") -> (value=w603:dbl)  [unwired: 1 in, 1 out]
        n172 = Logarithm Base 10(1:w603) -> (0:w602:dbl)
        n173 = Round To Nearest(number=w602) -> (nearest integer value=w601:dbl)
        n174 = Add(x=w601, y=11.0) -> (x+y=w599:dbl)
        n175 = To Unsigned Byte Integer(number=w599) -> (unsigned 8bit integer=w598:u8)
      }
      frame "drainrange" {
        (unwired) u8 11 items=["10fA  ", "100fA  ", "1nA  ", "10nA", "100nA", "1uA", "10uA", "100uA", "1mA", "10mA", "100mA", "1A"] ("Gate Range 2")
        n176 = Delete From Array(array=w636, index=0 ("Index")) -> (deleted portion=w627:string)  [unwired: 1 in, 1 out]
        n177 = Scan Value(string=w627, format string="") -> (value=w625:dbl)  [unwired: 1 in, 1 out]
        n178 = Logarithm Base 10(1:w625) -> (0:w624:dbl)
        n179 = Round To Nearest(number=w624) -> (nearest integer value=w623:dbl)
        n180 = Add(x=w623, y=11.0) -> (x+y=w621:dbl)
        n181 = To Unsigned Byte Integer(number=w621) -> (unsigned 8bit integer=w620:u8)
      }
      frame "drainrangemode" {
        n182 = Delete From Array(array=w650, index=0 ("Index")) -> (deleted portion=w651:string)  [unwired: 1 in, 1 out]
        n183 = case shown="\"f\"" w651 {
          tunnel: [w653 w654 w655] -> w640
          frame "a", Default {
            w653 = u16 0 items=["Auto", "Limited", "Fixed"] ("Gate Range\nmode 2")
          }
          frame "f" {
            w654 = u16 2 items=["Auto", "Limited", "Fixed"] ("Gate Range\nmode 2")
          }
          frame "l" {
            w655 = u16 1 items=["Auto", "Limited", "Fixed"] ("Gate Range\nmode 2")
          }
        }
      }
      frame "Error", Default {
      }
      frame "logfile" {
        n184 = Number To Decimal String(number=w670) -> (decimal integer string=w705:string)  [unwired: 1 in]
        n185 = Concatenate Strings(w704, "logfile" ("Substring"), w705, w668, ".txt" ("Substring")) -> (w702:string)
        n186 = String To Path(string=w702) -> (path=w675:path)
        n187 = Unbundle(w701) -> ("integration time"=w700:u32, "Short/Long integration time"=w699:dbl, "hold time (sec)"=w698:dbl, "delay time (sec)"=w697:dbl, "Step Time (0 disables)"=w696:dbl, "sweep method"=w695:u16, "Pulse period"=w694:dbl, "Base voltage"=w693:dbl, "Pulse width"=w692:dbl)
        n188 = Build Array(w700, w699, w698, w697, w696, w695, w694, w693, w692, w686, w687, w688, w689, w690, w691) -> (w679:dbl[])
        n189 = Insert Into Array(array=dbl[][] [] ("Input Array"), new element=w679) -> (w678:dbl[][])  [unwired: 2 in]
        n190 = call <vilib>:"compatOverwrite.vi"("overwrite (F)"=TRUE) -> ("overwrite?"=w673:T7)
        n191 = Open/Create/Replace File(file path (use dialog)=w675, error in=w677, operation (0:open)=w673) -> (refnum out=w683:refnum<file>, error out=w682:errorcluster)  [unwired: 3 in, 1 out]
        n192 = call "4155C Write array to file.vi"("Byte Stream File Refnum"=w683, "Header"=string[] ["Int Time", "Short/Long Itime", "Hold time", "Delay time", "Step time", "Sweep method", "Pulse period", "Base Voltage", "Pulse width", "Drain compliance", "Gate compliance", "Gate range mode", "Gate range", "S/D range mode", "S/D range"], "Data Array"=w678, "error in (no error)"=w682) -> ("dup refnum"=w685:refnum<file>, "error out"=w684:errorcluster)  [unwired: 1 in]
        n193 = Close File(refnum=w685, error in=w684) -> (error out=w676:errorcluster)  [unwired: 1 out]
      }
      frame "sample" {
        n194 = Number To Decimal String(number=w709) -> (decimal integer string=w757:string)  [unwired: 1 in]
        n195 = Fract/Exp String To Number(string=w754) -> (number=w715:dbl[])  [unwired: 3 in, 1 out]
        n196 = Concatenate Strings(w732, "-sample-" ("Substring"), w757, w707, ".txt" ("Substring")) -> (w755:string)
        n197 = String To Path(string=w755) -> (path=w736:path)
        n198 = Index Array(array=w715, index=0 ("Index")) -> (element=w752:dbl)
        n199 = Index Array(array=w715, index=2 ("Index")) -> (element=w748:dbl)
        n200 = Index Array(array=w715, index=3 ("Index")) -> (element=w717:dbl)
        n201 = Index Array(array=w715, index=4 ("Index")) -> (element=w714:dbl)
        n202 = call "4155C Config Sampling Measurements.vi"("Sampling interval"=w714, "Sample time"=w717, "Display on/off"=TRUE, "Timings"=w723, "Num Points"=w748, "error in (no error)"=w759, "Drain Compliance"=w758, "Gate Compliance"=w733, "VISA session"=w760) -> ("error out"=w761:errorcluster, "dup VISA resource name"=w762:refnum<visa-resource-name>)  [unwired: 1 in]
        n203 = Index Array(array=w715, index=1 ("Index")) -> (element=w749:dbl)
        n204 = call "4155C Take Sample.vi"("Emergency Stop"=w729, "error in (no error)"=w761, "Vd"=w749, "Vg"=w752, "VISA resource name in"=w762) -> ("error out"=w727:errorcluster, "Id"=w764:dbl[], "Ig"=w738:dbl[], "VISA Resource Name out"=w725:refnum<visa-resource-name>, "Is"=w763:dbl[], "Time"=w742:dbl[])  [unwired: 1 in]
        n205 = Insert Into Array(array=dbl[][] [] ("Input Array"), new element=w742) -> (w741:dbl[][])  [unwired: 2 in]
        n206 = Insert Into Array(array=w741, new element=w738) -> (w740:dbl[][])  [unwired: 2 in]
        n207 = Insert Into Array(array=w740, new element=w764) -> (w739:dbl[][])  [unwired: 2 in]
        n208 = VISA Write(VISA resource name=w725, write buffer=":DISP ON" ("write buffer (\"\")"), error in (no error)=w727) -> (VISA resource name out=w724:refnum<visa-resource-name>, error out=w726:errorcluster)  [unwired: 1 out]
        n209 = Insert Into Array(array=w739, new element=w763) -> (w731:dbl[][])  [unwired: 2 in]
        n210 = Transpose 2D Array(2D array=w731) -> (transposed array=w730:dbl[][])
        n211 = call <vilib>:"compatOverwrite.vi"("overwrite (F)"=TRUE) -> ("overwrite?"=w712:T7)
        n212 = Open/Create/Replace File(file path (use dialog)=w736, error in=w726, operation (0:open)=w712) -> (refnum out=w745:refnum<file>, error out=w744:errorcluster)  [unwired: 3 in, 1 out]
        n213 = call "4155C Write array to file.vi"("Byte Stream File Refnum"=w745, "Header"=string[] ["Time /s", "Ig /A", "Id /A", "Is /A"], "Data Array"=w730, "error in (no error)"=w744) -> ("dup refnum"=w747:refnum<file>, "error out"=w746:errorcluster)  [unwired: 1 in]
        n214 = Close File(refnum=w747, error in=w746) -> (error out=w734:errorcluster)  [unwired: 1 out]
      }
      frame "samplei" {
        n215 = Number To Decimal String(number=w766) -> (decimal integer string=w818:string)  [unwired: 1 in]
        n216 = Fract/Exp String To Number(string=w815) -> (number=w782:dbl[])  [unwired: 3 in, 1 out]
        n217 = Concatenate Strings(w797, "-samplei-" ("Substring"), w818, w765, ".txt" ("Substring")) -> (w816:string)
        n218 = String To Path(string=w816) -> (path=w800:path)
        n219 = Index Array(array=w782, index=4 ("Index")) -> (element=w776:dbl)
        n220 = Index Array(array=w782, index=3 ("Index")) -> (element=w777:dbl)
        n221 = Index Array(array=w782, index=1 ("Index")) -> (element=w779:dbl)
        n222 = Index Array(array=w782, index=0 ("Index")) -> (element=w780:dbl)
        n223 = Index Array(array=w782, index=2 ("Index")) -> (element=w778:dbl)
        n224 = call "4155C Config SamplingI Measurements.vi"("Sample time"=w778, "Display on/off"=TRUE, "Timings"=w789, "Num Points"=w779, "error in (no error)"=w820, "Sampling interval"=w777, "VISA session"=w821) -> ("error out"=w822:errorcluster, "dup VISA resource name"=w823:refnum<visa-resource-name>)  [unwired: 3 in]
        n225 = call "4155C Take SampleI.vi"("Emergency Stop"=w794, "error in (no error)"=w822, "Idg 2"=w780, "Vdg compliance 2"=w776, "VISA resource name in"=w823) -> ("error out"=w792:errorcluster, "Idg"=w825:dbl[], "Vdg"=w802:dbl[], "VISA Resource Name out"=w790:refnum<visa-resource-name>, "Is"=w824:dbl[], "Time"=w806:dbl[])  [unwired: 1 in]
        n226 = Insert Into Array(array=dbl[][] [] ("Input Array"), new element=w806) -> (w805:dbl[][])  [unwired: 2 in]
        n227 = Insert Into Array(array=w805, new element=w802) -> (w804:dbl[][])  [unwired: 2 in]
        n228 = Insert Into Array(array=w804, new element=w825) -> (w803:dbl[][])  [unwired: 2 in]
        n229 = VISA Write(VISA resource name=w790, write buffer=":DISP ON" ("write buffer (\"\")"), error in (no error)=w792) -> (VISA resource name out=w775:refnum<visa-resource-name>, error out=w791:errorcluster)  [unwired: 1 out]
        n230 = Insert Into Array(array=w803, new element=w824) -> (w796:dbl[][])  [unwired: 2 in]
        n231 = Transpose 2D Array(2D array=w796) -> (transposed array=w795:dbl[][])
        n232 = call <vilib>:"compatOverwrite.vi"("overwrite (F)"=TRUE) -> ("overwrite?"=w770:T7)
        n233 = Open/Create/Replace File(file path (use dialog)=w800, error in=w791, operation (0:open)=w770) -> (refnum out=w809:refnum<file>, error out=w808:errorcluster)  [unwired: 3 in, 1 out]
        n234 = call "4155C Write array to file.vi"("Byte Stream File Refnum"=w809, "Header"=string[] ["Time /s", "Vdg /V", "Idg /A", "Is /A"], "Data Array"=w795, "error in (no error)"=w808) -> ("dup refnum"=w811:refnum<file>, "error out"=w810:errorcluster)  [unwired: 1 in]
        n235 = Close File(refnum=w811, error in=w810) -> (error out=w773:errorcluster)  [unwired: 1 out]
        n236 = VISA Write(VISA resource name=w775, write buffer=";:PAGE:SCON:STAN OFF;:PAGE:CHAN:VSU2:DIS;" ("write buffer (\"\")"), error in (no error)=w773) -> (VISA resource name out=w771:refnum<visa-resource-name>, error out=w772:errorcluster)  [unwired: 1 out]
      }
      frame "#" {
        n237 = VISA Write(VISA resource name=w832, write buffer=":DISP ON" ("write buffer (\"\")"), error in (no error)=w831) -> (VISA resource name out=w830:refnum<visa-resource-name>, error out=w829:errorcluster)  [unwired: 1 out]
      }
      frame "stressV" {
        n238 = Number To Decimal String(number=w842) -> (decimal integer string=w883:string)  [unwired: 1 in]
        n239 = Fract/Exp String To Number(string=w880) -> (number=w853:dbl[])  [unwired: 3 in, 1 out]
        n240 = Concatenate Strings(w867, "-stressV-" ("Substring"), w883, w841, ".txt" ("Substring")) -> (w881:string)
        n241 = String To Path(string=w881) -> (path=w871:path)
        n242 = Index Array(array=w853, index=3 ("Index")) -> (element=w850:dbl)
        n243 = Index Array(array=w853, index=1 ("Index")) -> (element=w848:dbl)
        n244 = Index Array(array=w853, index=0 ("Index")) -> (element=w847:dbl)
        n245 = Index Array(array=w853, index=4 ("Index")) -> (element=w852:dbl)
        n246 = Index Array(array=w853, index=2 ("Index")) -> (element=w849:dbl)
        n247 = call "4155C Config V Stress.vi"("VISA session"=w886, "ID compliance"=w850, "VD"=w848, "VG"=w847, "IG compliance"=w849, "error in (no error)"=w885, "Display on/off"=TRUE) -> ("dup VISA resource name"=w888:refnum<visa-resource-name>, "error out"=w887:errorcluster)
        n248 = call "4155C Apply Stress.vi"("error in (no error)"=w887, "Duration"=w852, "Emergency Stop"=w866, "VISA resource name in"=w888) -> ("error out"=w864:errorcluster, "VISA Resource Name out"=w862:refnum<visa-resource-name>)
        n249 = VISA Write(VISA resource name=w862, write buffer=":DISP ON" ("write buffer (\"\")"), error in (no error)=w864) -> (VISA resource name out=w861:refnum<visa-resource-name>, error out=w863:errorcluster)  [unwired: 1 out]
        n250 = call <vilib>:"compatOverwrite.vi"("overwrite (F)"=TRUE) -> ("overwrite?"=w846:T7)
        n251 = Open/Create/Replace File(file path (use dialog)=w871, error in=w863, operation (0:open)=w846) -> (refnum out=w874:refnum<file>, error out=w873:errorcluster)  [unwired: 3 in, 1 out]
        n252 = call "4155C Write array to file.vi"("Byte Stream File Refnum"=w874, "Header"=string[] ["V stress completed successfully", ""], "error in (no error)"=w873) -> ("dup refnum"=w876:refnum<file>, "error out"=w875:errorcluster)  [unwired: 2 in]
        n253 = Close File(refnum=w876, error in=w875) -> (error out=w869:errorcluster)  [unwired: 1 out]
      }
      frame "stressI" {
        n254 = Number To Decimal String(number=w890) -> (decimal integer string=w927:string)  [unwired: 1 in]
        n255 = Fract/Exp String To Number(string=w924) -> (number=w899:dbl[])  [unwired: 3 in, 1 out]
        n256 = Concatenate Strings(w911, "-stressI-" ("Substring"), w927, w889, ".txt" ("Substring")) -> (w925:string)
        n257 = String To Path(string=w925) -> (path=w915:path)
        n258 = Index Array(array=w899, index=1 ("Index")) -> (element=w895:dbl)
        n259 = Index Array(array=w899, index=0 ("Index")) -> (element=w896:dbl)
        n260 = call "4155C Config I Stress.vi"("VISA session"=w930, "IDG"=w896, "VDG compliance"=w895, "error in (no error)"=w929, "Display on/off"=TRUE) -> ("dup VISA resource name"=w932:refnum<visa-resource-name>, "error out"=w931:errorcluster)
        n261 = Index Array(array=w899, index=2 ("Index")) -> (element=w897:dbl)
        n262 = call "4155C Apply Stress.vi"("error in (no error)"=w931, "Duration"=w897, "Emergency Stop"=w910, "VISA resource name in"=w932) -> ("error out"=w908:errorcluster, "VISA Resource Name out"=w906:refnum<visa-resource-name>)
        n263 = VISA Write(VISA resource name=w906, write buffer=":DISP ON" ("write buffer (\"\")"), error in (no error)=w908) -> (VISA resource name out=w905:refnum<visa-resource-name>, error out=w907:errorcluster)  [unwired: 1 out]
        n264 = call <vilib>:"compatOverwrite.vi"("overwrite (F)"=TRUE) -> ("overwrite?"=w894:T7)
        n265 = Open/Create/Replace File(file path (use dialog)=w915, error in=w907, operation (0:open)=w894) -> (refnum out=w918:refnum<file>, error out=w917:errorcluster)  [unwired: 3 in, 1 out]
        n266 = call "4155C Write array to file.vi"("Byte Stream File Refnum"=w918, "Header"=string[] ["I stress completed successfully", ""], "error in (no error)"=w917) -> ("dup refnum"=w920:refnum<file>, "error out"=w919:errorcluster)  [unwired: 2 in]
        n267 = Close File(refnum=w920, error in=w919) -> (error out=w913:errorcluster)  [unwired: 1 out]
      }
      frame "vsu2pulse" {
        n268 = Number To Decimal String(number=w934) -> (decimal integer string=w969:string)  [unwired: 1 in]
        n269 = Fract/Exp String To Number(string=w966) -> (number=w942:dbl[])  [unwired: 3 in, 1 out]
        n270 = Concatenate Strings(w954, "-vsu2-" ("Substring"), w969, w933, ".txt" ("Substring")) -> (w967:string)
        n271 = String To Path(string=w967) -> (path=w958:path)
        n272 = Index Array(array=w942, index=1 ("Index")) -> (element=w941:dbl)
        n273 = Index Array(array=w942, index=0 ("Index")) -> (element=w939:dbl)
        n274 = call "4155C Config VSU2 Stress.vi"("error in (no error)"=w971, "VSU2"=w939, "Display on/off"=TRUE, "VISA session"=w972) -> ("error out"=w973:errorcluster, "dup VISA resource name"=w974:refnum<visa-resource-name>)
        n275 = call "4155C Apply Stress.vi"("error in (no error)"=w973, "Duration"=w941, "Emergency Stop"=w953, "VISA resource name in"=w974) -> ("error out"=w951:errorcluster, "VISA Resource Name out"=w949:refnum<visa-resource-name>)
        n276 = VISA Write(VISA resource name=w949, write buffer=":DISP ON" ("write buffer (\"\")"), error in (no error)=w951) -> (VISA resource name out=w948:refnum<visa-resource-name>, error out=w950:errorcluster)  [unwired: 1 out]
        n277 = call <vilib>:"compatOverwrite.vi"("overwrite (F)"=TRUE) -> ("overwrite?"=w938:T7)
        n278 = Open/Create/Replace File(file path (use dialog)=w958, error in=w950, operation (0:open)=w938) -> (refnum out=w961:refnum<file>, error out=w960:errorcluster)  [unwired: 3 in, 1 out]
        n279 = call "4155C Write array to file.vi"("Byte Stream File Refnum"=w961, "Header"=string[] ["VSU2 pulse completed successfully", ""], "error in (no error)"=w960) -> ("dup refnum"=w963:refnum<file>, "error out"=w962:errorcluster)  [unwired: 2 in]
        n280 = Close File(refnum=w963, error in=w962) -> (error out=w956:errorcluster)  [unwired: 1 out]
      }
      frame "sample-fpp" {
        w987 = string[] ["Time /s", "Id VgVd /A", "Ig VgVd /A", "Vp1 VgVd /V", "Vp2 VgVd /V"] ("Header")
        w991 = "%d" ("format string")
        n281 = Number To Decimal String(number=w976) -> (decimal integer string=w1039:string)  [unwired: 1 in]
        n282 = Fract/Exp String To Number(string=w1036) -> (number=w1024:dbl[])  [unwired: 3 in, 1 out]
        n283 = Concatenate Strings(w1030, "-samplefpp-" ("Substring"), w1039, w975, ".txt" ("Substring")) -> (w1037:string)
        n284 = String To Path(string=w1037) -> (path=w999:path)
        n285 = Index Array(array=w1024, index=0 ("Index")) -> (element=w985:dbl)
        n286 = Index Array(array=w1024, index=1 ("Index")) -> (element=w984:dbl)
        n287 = Index Array(array=w1024, index=2 ("Index")) -> (element=w1032:dbl)
        n288 = Index Array(array=w1024, index=3 ("Index")) -> (element=w1022:dbl)
        n289 = call "4155C Config Sampling Measurements FPP.vi"("VISA session"=w1042, "Num Points"=w1032, "Vg"=w985, "Display on/off"=TRUE, "Gate Compliance"=w1031, "Drain Compliance"=w1040, "Standby"="Standby", "error in (no error)"=w1041, "Timings"=w1029, "Vd"=w984, "Sample time"=w1022) -> ("dup VISA resource name"=w1001:refnum<visa-resource-name>, "error out"=w1000:errorcluster)  [unwired: 3 in]
        n290 = Number To Decimal String(number=w985) -> (decimal integer string=w1011:string)  [unwired: 1 in]
        n291 = call "4155C Take Sample FPP.vi"("VISA resource name in"=w1001, "error in (no error)"=w1000, "Emergency Stop"=w1002) -> ("Time"=w1006:dbl[], "Vp1"=w1016:dbl[], "VISA Resource Name out"=w982:refnum<visa-resource-name>, "Ig"=w1004:dbl[], "Id"=w1005:dbl[], "Vp2"=w1014:dbl[], "error out"=w1003:errorcluster)  [unwired: 10 in]
        n292 = Insert Into Array(array=dbl[][] [] ("Input Array"), new element=w1006) -> (w1020:dbl[][])  [unwired: 2 in]
        n293 = Number To Decimal String(number=w984) -> (decimal integer string=w1009:string)  [unwired: 1 in]
        n294 = Insert Into Array(array=w1020, new element=w1005) -> (w1019:dbl[][])  [unwired: 2 in]
        n295 = Concatenate Strings("(Vg = " ("Substring"), w1011, "V, Vd = " ("Substring"), w1009, "V)" ("Substring")) -> (w1007:string)
        n296 = Insert Into Array(array=w1019, new element=w1004) -> (w1018:dbl[][])  [unwired: 2 in]
        n297 = Insert Into Array(array=w1018, new element=w1016) -> (w1015:dbl[][])  [unwired: 2 in]
        n298 = Insert Into Array(array=w1015, new element=w1014) -> (w983:dbl[][])  [unwired: 2 in]
        n299 = call <vilib>:"compatOverwrite.vi"("overwrite (F)"=TRUE) -> ("overwrite?"=w980:T7)
        n300 = Open/Create/Replace File(file path (use dialog)=w999, error in=w1003, operation (0:open)=w980) -> (refnum out=w996:refnum<file>, error out=w997:errorcluster)  [unwired: 3 in, 1 out]
        n301 = Array To Spreadsheet String(array=w987, 3:w991) -> (spreadsheet string=w993:string)  [unwired: 1 in]
        n302 = Transpose 2D Array(2D array=w983) -> (transposed array=w1013:dbl[][])
        n303 = Search and Replace String(replace all?=TRUE ("replace all? (F)"), input string=w993, search string="VgVd", replace string=w1007) -> (result string=w989:string)  [unwired: 4 in, 3 out]
        n304 = Spreadsheet String To Array(format string=w991, spreadsheet string=w989, array type (2D Dbl)=w987) -> (array=w988:string[])  [unwired: 1 in]
        n305 = call "4155C Write array to file.vi"("Byte Stream File Refnum"=w996, "Header"=w988, "Data Array"=w1013, "error in (no error)"=w997) -> ("dup refnum"=w994:refnum<file>, "error out"=w995:errorcluster)  [unwired: 1 in]
        n306 = Close File(refnum=w994, error in=w995) -> (error out=w981:errorcluster)  [unwired: 1 out]
      }
      frame "resample-fpp" {
        w1057 = string[] ["Time /s", "Id VgVd /A", "Ig VgVd /A", "Vp1 VgVd /V", "Vp2 VgVd /V"] ("Header")
        w1061 = "%d" ("format string")
        n307 = Number To Decimal String(number=w1043) -> (decimal integer string=w1101:string)  [unwired: 1 in]
        n308 = Fract/Exp String To Number(string=w1098) -> (number=w1050:dbl[])  [unwired: 3 in, 1 out]
        n309 = Concatenate Strings(w1094, "-resamplefpp-" ("Substring"), w1101, w1044, ".txt" ("Substring")) -> (w1099:string)
        n310 = String To Path(string=w1099) -> (path=w1069:path)
        n311 = Index Array(array=w1050, index=0 ("Index")) -> (element=w1056:dbl)
        n312 = Index Array(array=w1050, index=1 ("Index")) -> (element=w1055:dbl)
        n313 = Number To Decimal String(number=w1056) -> (decimal integer string=w1079:string)  [unwired: 1 in]
        n314 = call "4155C Take Sample FPP.vi"("VISA resource name in"=w1052, "error in (no error)"=w1051, "Emergency Stop"=w1070) -> ("Time"=w1074:dbl[], "Vp1"=w1084:dbl[], "VISA Resource Name out"=w1054:refnum<visa-resource-name>, "Ig"=w1072:dbl[], "Id"=w1073:dbl[], "Vp2"=w1082:dbl[], "error out"=w1071:errorcluster)  [unwired: 10 in]
        n315 = Insert Into Array(array=dbl[][] [] ("Input Array"), new element=w1074) -> (w1088:dbl[][])  [unwired: 2 in]
        n316 = Number To Decimal String(number=w1055) -> (decimal integer string=w1077:string)  [unwired: 1 in]
        n317 = Insert Into Array(array=w1088, new element=w1073) -> (w1087:dbl[][])  [unwired: 2 in]
        n318 = Concatenate Strings("(Vg = " ("Substring"), w1079, "V, Vd = " ("Substring"), w1077, "V)" ("Substring")) -> (w1075:string)
        n319 = Insert Into Array(array=w1087, new element=w1072) -> (w1086:dbl[][])  [unwired: 2 in]
        n320 = Insert Into Array(array=w1086, new element=w1084) -> (w1083:dbl[][])  [unwired: 2 in]
        n321 = Insert Into Array(array=w1083, new element=w1082) -> (w1049:dbl[][])  [unwired: 2 in]
        n322 = call <vilib>:"compatOverwrite.vi"("overwrite (F)"=TRUE) -> ("overwrite?"=w1048:T7)
        n323 = Open/Create/Replace File(file path (use dialog)=w1069, error in=w1071, operation (0:open)=w1048) -> (refnum out=w1066:refnum<file>, error out=w1067:errorcluster)  [unwired: 3 in, 1 out]
        n324 = Array To Spreadsheet String(array=w1057, 3:w1061) -> (spreadsheet string=w1063:string)  [unwired: 1 in]
        n325 = Transpose 2D Array(2D array=w1049) -> (transposed array=w1081:dbl[][])
        n326 = Search and Replace String(replace all?=TRUE ("replace all? (F)"), input string=w1063, search string="VgVd", replace string=w1075) -> (result string=w1059:string)  [unwired: 4 in, 3 out]
        n327 = Spreadsheet String To Array(format string=w1061, spreadsheet string=w1059, array type (2D Dbl)=w1057) -> (array=w1058:string[])  [unwired: 1 in]
        n328 = call "4155C Write array to file.vi"("Byte Stream File Refnum"=w1066, "Header"=w1058, "Data Array"=w1081, "error in (no error)"=w1067) -> ("dup refnum"=w1064:refnum<file>, "error out"=w1065:errorcluster)  [unwired: 1 in]
        n329 = Close File(refnum=w1064, error in=w1065) -> (error out=w1053:errorcluster)  [unwired: 1 out]
      }
      frame "serial" {
        n330 = Index Array(array=w1104, index=0 ("Index")) -> (element=w1103:string)
        n331 = call "Serial write and read v0.2.vi"("Termination char\n(0xA = '\\n' = LF)\n(0xD = '\\r' = CR)"="Termination char\n(0xA = '\\n' = LF)\n(0xD = '\\r' = CR)", "Enable Termination\nChar (T)"="Enable Termination\nChar (T)", "parity"="parity", "stop bits"="stop bits", "string to write"=w1103, "flow control"="flow control", "bytes to read"="bytes to read", "Serial Settings:Serial End Mode for Reads"="Serial Settings:Serial End Mode for Reads", "Timeout (ms)"="Timeout (ms)", "error in (no error)"=w1109, "VISA resource name"="VISA resource name", "baud rate"="baud rate", "data bits"="data bits") -> ("read string"=→"Serial output":string, "error out"=w1108:errorcluster)  [unwired: 1 in]
      }
    }
  }
  "error out" <- w2
